vi "数据表比对.vi"(8 "error in (no error)":errorcluster, 9 "查询元素输入":string(combo), 10 "仪器日志参数":string, 11 "table输入":string(combo)) -> (0 "error out":errorcluster, 1 "columns输出":string[](array[string]), 2 "待发送第一条数据":string[](array[string]), 3 "待发送数据":string[][](table))   [LabVIEW 2016, in "数据传输系统.lvlib"]
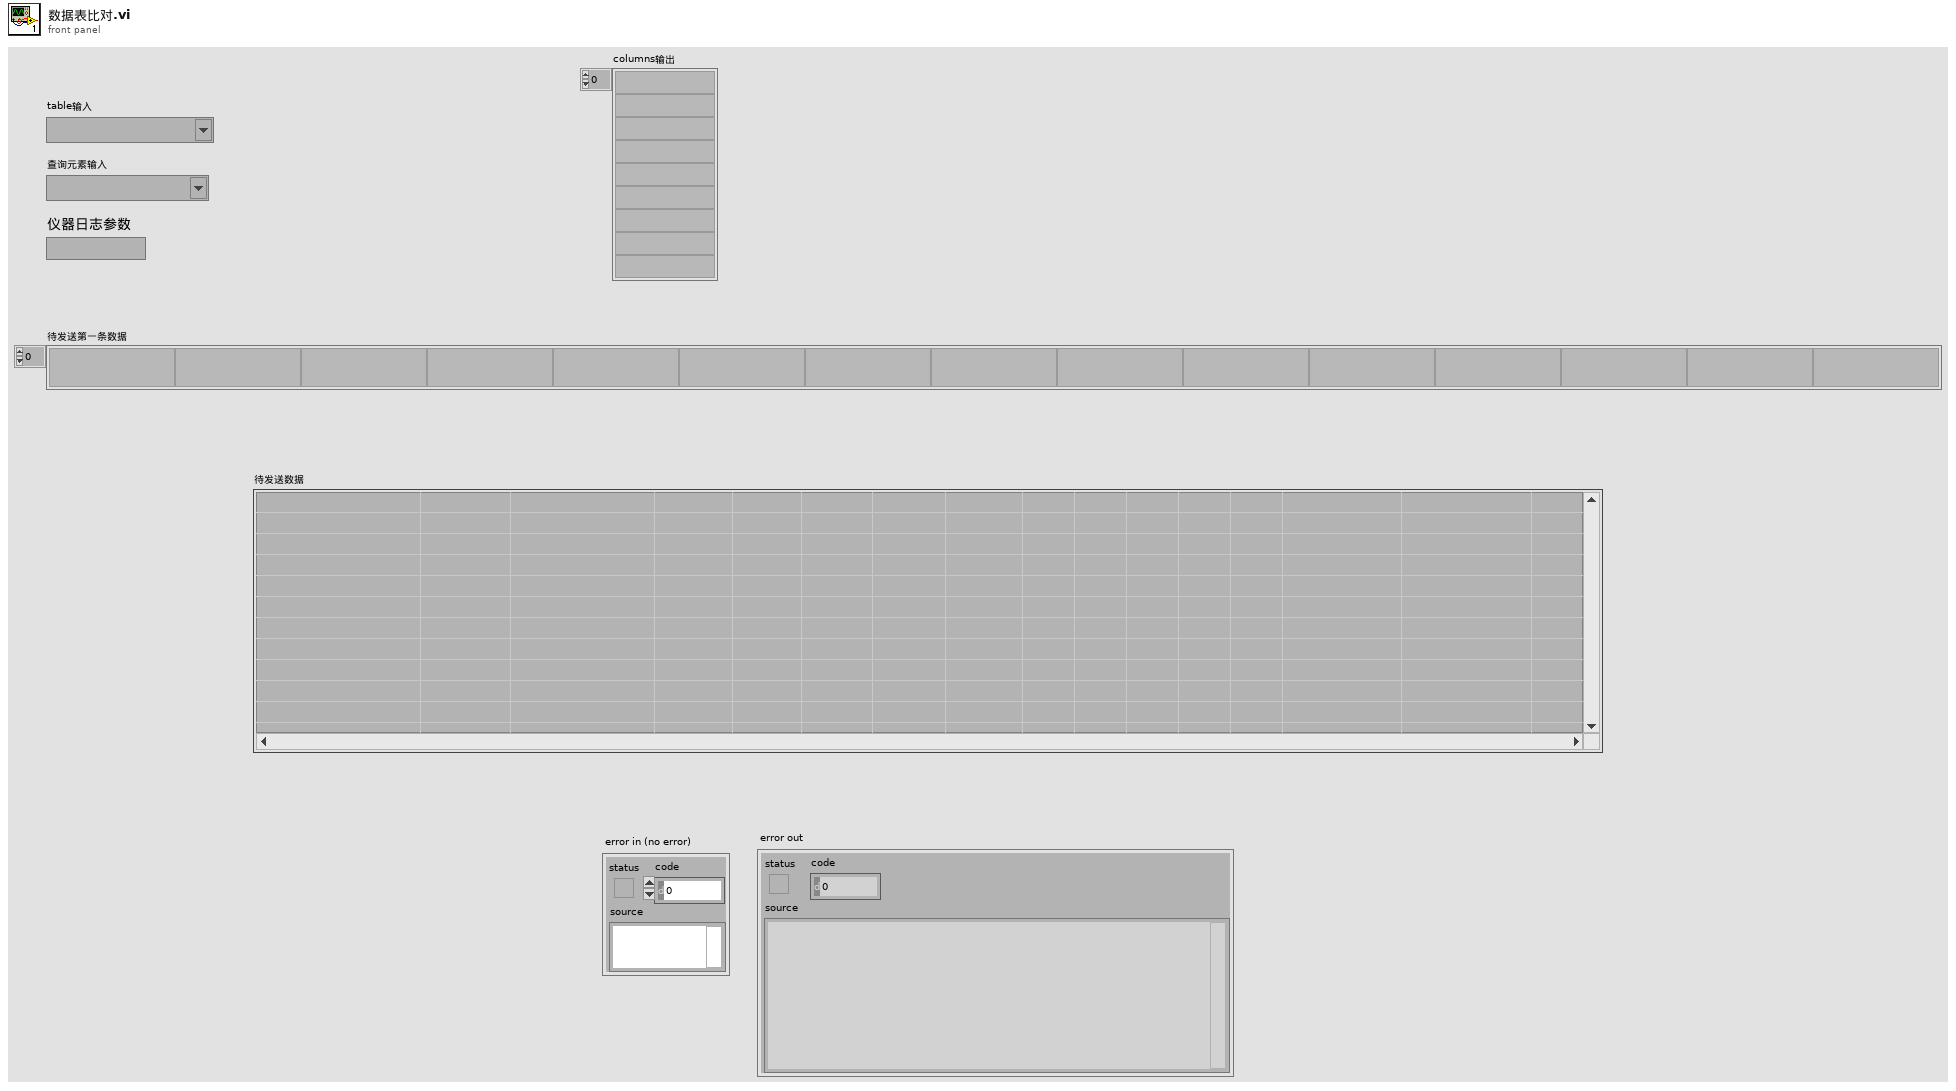
[diagram p1: front panel]
types:
  T1 = cluster{"氨氮仪器日志索引起始时间":string, "总磷仪器日志索引起始时间":string, "总氮仪器日志索引起始时间":string, "CODMn仪器日志索引起始时间":string, "CODCr仪器日志索引起始时间":string, "系统仪器日志索引起始时间":string}
  T2 = cluster{"氨氮仪器参数索引起始时间":string, "总磷仪器参数索引起始时间":string, "总氮仪器参数索引起始时间":string, "CODMn仪器参数索引起始时间":string, "CODCr仪器参数索引起始时间":string, "DO仪器参数索引起始时间":string, "PH仪器参数索引起始时间":string, "比电导率仪器参数索引起始时间":string, "水温仪器参数索引起始时间":string, "浊度仪器参数索引起始时间":string, "叶绿素a仪器参数索引起始时间":string, "藻密度仪器参数索引起始时间":string, "ORP仪器参数索引起始时间":string}
  T3 = cluster{"氨氮报警信息索引起始时间":string, "总磷报警信息索引起始时间":string, "总氮报警信息索引起始时间":string, "CODMn报警信息索引起始时间":string, "CODCr报警信息索引起始时间":string, "DO报警信息索引起始时间":string, "PH报警信息索引起始时间":string, "比电导率报警信息索引起始时间":string, "水温报警信息索引起始时间":string, "浊度报警信息索引起始时间":string, "叶绿素报警信息索引起始时间":string, "系统报警信息索引起始时间":string}
  T4 = cluster{"氨氮零点核查索引起始时间":string, "总磷零点核查索引起始时间":string, "总氮零点核查索引起始时间":string, "CODMn零点核查索引起始时间":string, "CODCr零点核查索引起始时间":string, "亚硝酸盐零点核查索引起始时间":string, "硫化物零点核查索引起始时间":string, "ORP零点核查索引起始时间":string}
  T5 = cluster{"氨氮标样核查索引起始时间":string, "总磷标样核查索引起始时间":string, "总氮标样核查索引起始时间":string, "CODMn标样核查索引起始时间":string, "CODCr标样核查索引起始时间":string, "DO标样核查索引起始时间":string, "PH标样核查索引起始时间":string, "比电导率标样核查索引起始时间":string, "水温标样核查索引起始时间":string, "浊度标样核查索引起始时间":string, "叶绿素a标样核查索引起始时间":string, "藻密度标样核查索引起始时间":string, "亚硝酸盐标样核查索引起始时间":string, "硫化物标样核查索引起始时间":string, "ORP标样核查索引起始时间":string}
  T6 = cluster{"氨氮跨度核查索引起始时间":string, "总磷跨度核查索引起始时间":string, "总氮跨度核查索引起始时间":string, "CODMn跨度核查索引起始时间":string, "CODCr跨度核查索引起始时间":string, "亚硝酸盐跨度核查索引起始时间":string, "硫化物跨度核查索引起始时间":string, "ORP跨度核查索引起始时间":string}
  T7 = typedef "LVDateTimeRec.ctl" = cluster{"秒数的小数部分":dbl, "秒":i32, "分":i32, "时":i32, "日":i32, "月":i32, "年":i32, "天数（周）":i32, "天数（年）":i32, "DST":i32}
  T8 = cluster{"氨氮加标回收索引起始时间":string, "总磷加标回收索引起始时间":string, "总氮加标回收索引起始时间":string, "CODMn加标回收索引起始时间":string, "CODCr加标回收索引起始时间":string}
  T9 = cluster{"氨氮平行样索引起始时间":string, "总磷平行样索引起始时间":string, "总氮平行样索引起始时间":string, "CODMn平行样索引起始时间":string, "CODCr平行样索引起始时间":string}
  T10 = cluster{"氨氮集成干预索引起始时间":string, "总磷集成干预索引起始时间":string, "总氮集成干预索引起始时间":string, "CODMn集成干预索引起始时间":string, "CODCr集成干预索引起始时间":string, "DO集成干预索引起始时间":string, "PH集成干预索引起始时间":string, "比电导率集成干预索引起始时间":string, "水温集成干预索引起始时间":string, "浊度集成干预索引起始时间":string, "叶绿素a集成干预索引起始时间":string, "藻密度集成干预索引起始时间":string, "亚硝酸盐集成干预索引起始时间":string, "硫化物集成干预索引起始时间":string, "ORP集成干预索引起始时间":string}
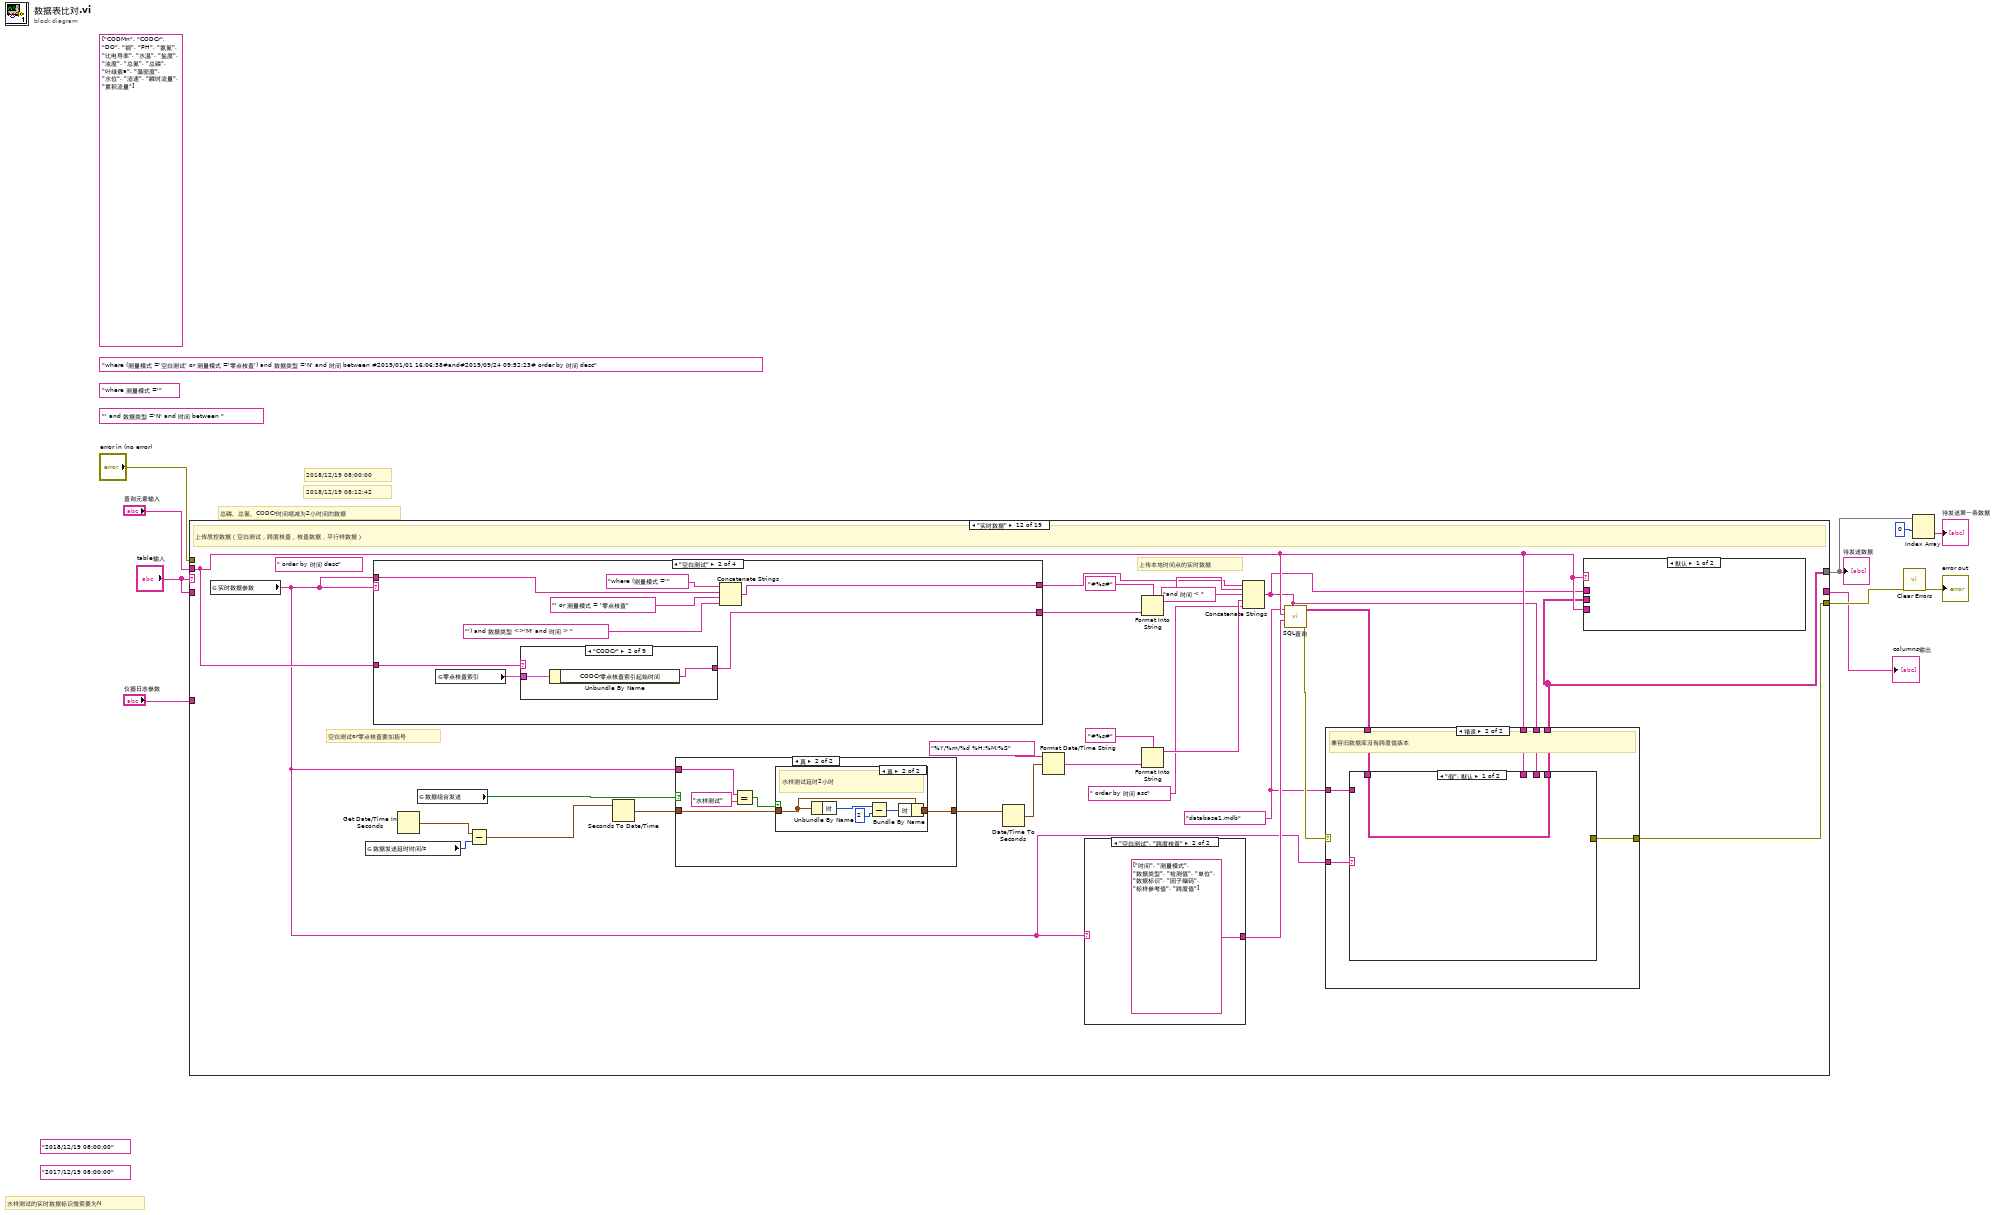
[diagram p0: block diagram]
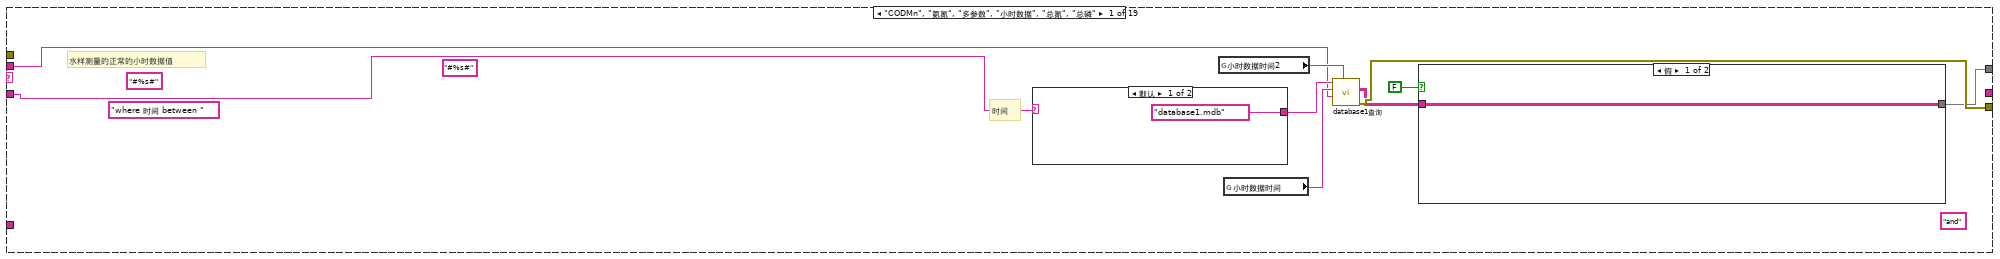
[diagram p2: hidden frame]
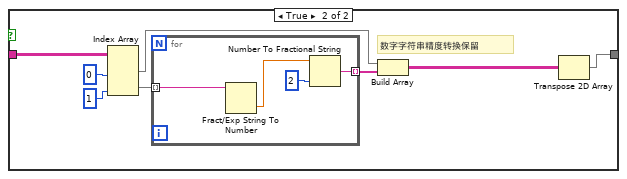
[diagram p3: hidden frame]
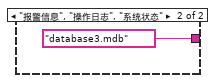
[diagram p4: hidden frame]
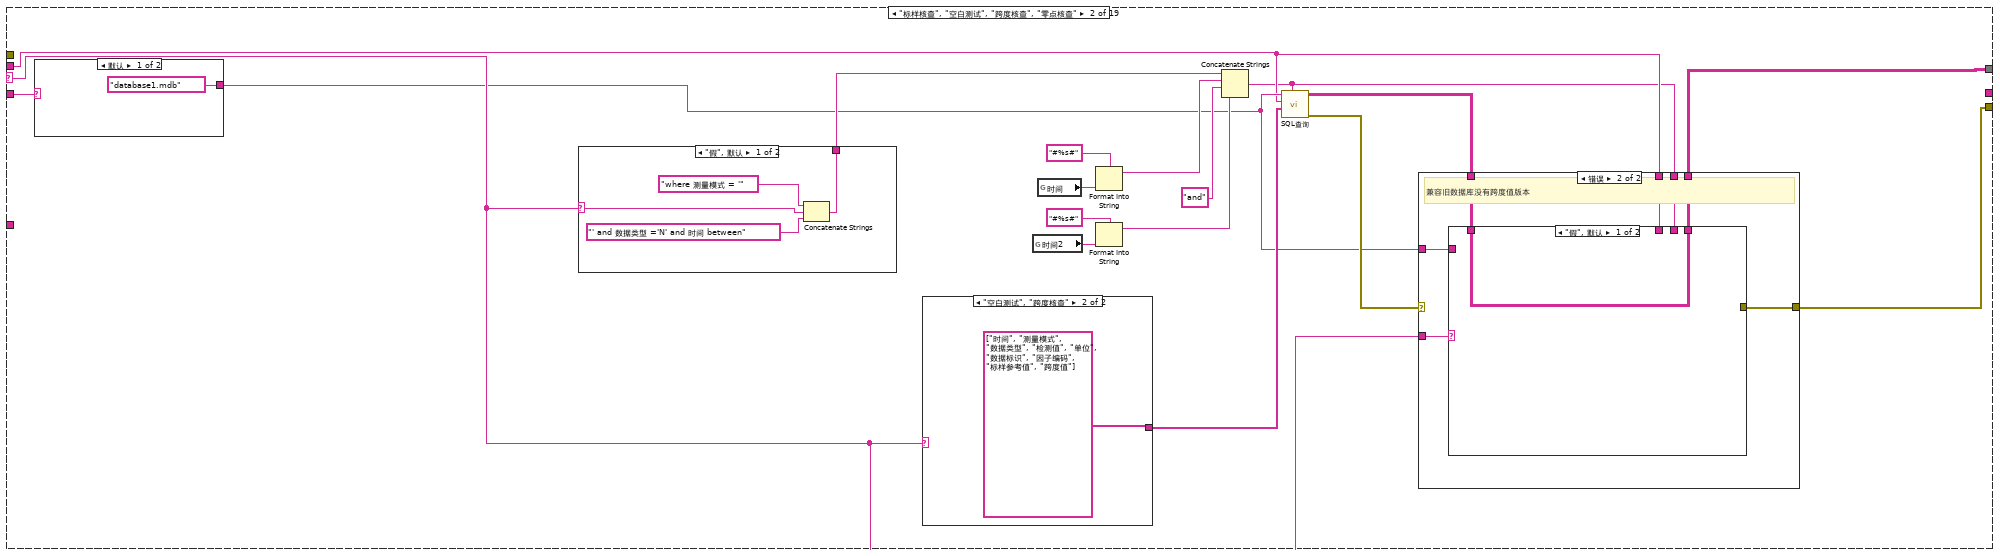
[diagram p5: hidden frame]
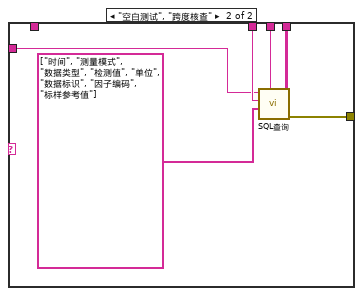
[diagram p7: hidden frame]
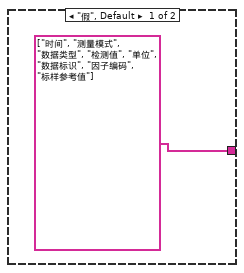
[diagram p8: hidden frame]
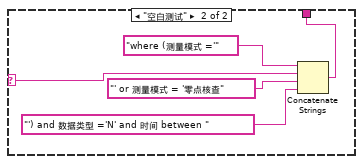
[diagram p9: hidden frame]
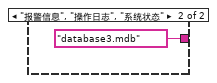
[diagram p10: hidden frame]
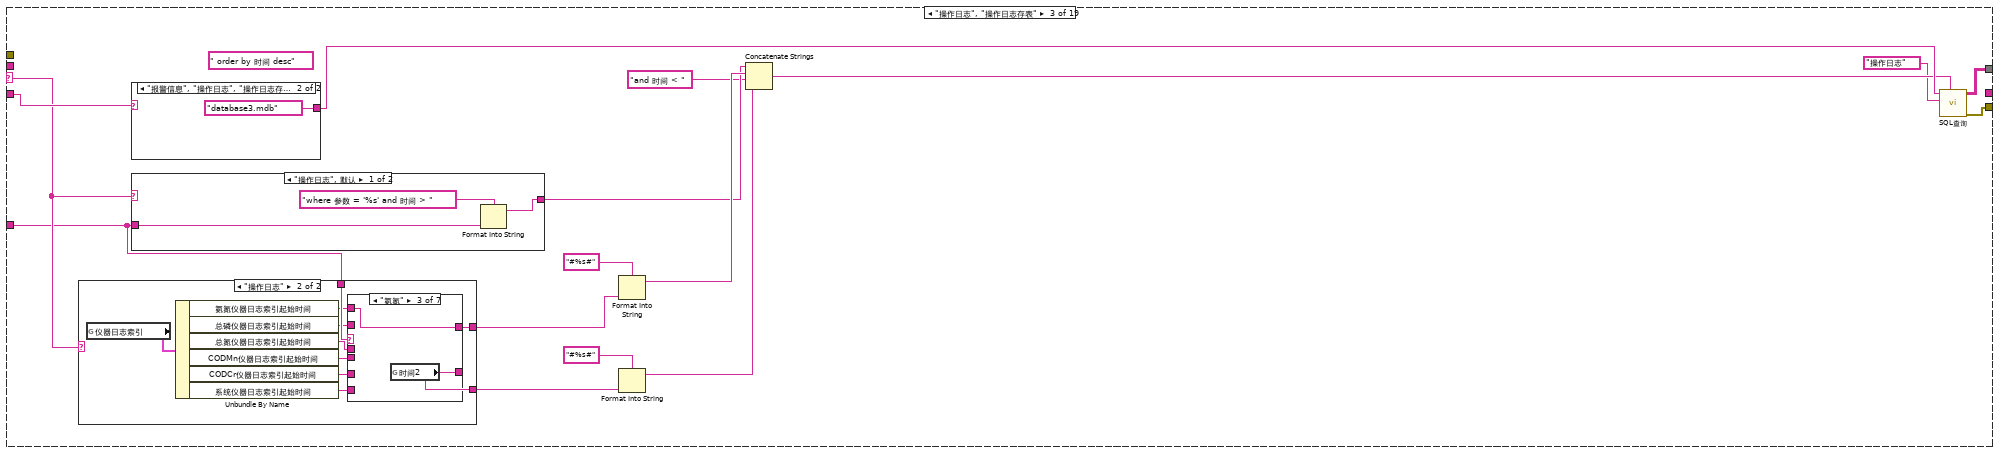
[diagram p11: hidden frame]
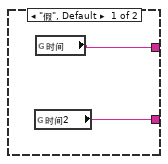
[diagram p12: hidden frame]
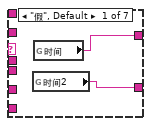
[diagram p13: hidden frame]
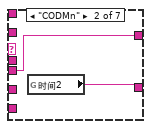
[diagram p14: hidden frame]
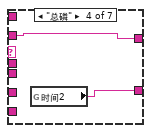
[diagram p15: hidden frame]
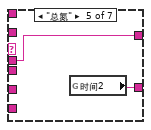
[diagram p16: hidden frame]
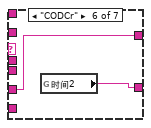
[diagram p17: hidden frame]
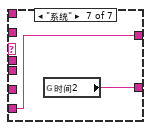
[diagram p18: hidden frame]
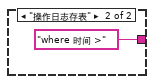
[diagram p19: hidden frame]
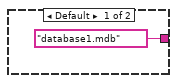
[diagram p20: hidden frame]
diagram:
  (unwired) "' and 数据类型 ='N' and 时间 between "
  (unwired) "where 测量模式 ='" ("condition")
  (unwired) "where (测量模式 ='空白测试' or 测量模式 ='零点核查') and 数据类型 ='N' and 时间 between #2019/01/01 16:06:38#and#2019/09/24 09:52:23# order by 时间 desc" ("condition")
  (unwired) string[] ["CODMn", "CODCr", "DO", "铜", "PH", "氨氮", "比电导率", "水温", "盐度", "浊度", "总氮", "总磷", "叶绿素a", "藻密度", "水位", "流速", "瞬时流量", "累积流量"] ("查询参数数组")
  (unwired) "2017/12/19 08:00:00"
  (unwired) "2018/12/19 08:00:00"
  # "水样测试的实时数据标识搜索要为N"
  # "2018/12/19 08:00:00"
  # "总磷、总氮、CODCr时间缩减为2小时间的数据"
  # "2018/12/19 08:12:42"
  n1 = case shown="\"实时数据\"" "table输入" {
    selector: "table输入" -> [_ w41 w86 _ _ _ _ w314 _ _ _ _ _ _ _ _ _ _ _]
    tunnel: "error in (no error)" -> [_ _ _ _ _ _ _ _ _ _ w418 _ _ _ _ _ _ _ _]
    tunnel: [w17 w35 w95 w144 w150 w202 w294 w328 w408 w415 w418 w419 w600 w661 w724 w788 w829 w872 w920] -> w8
    tunnel: [w13 w36 w93 w142 w178 w204 w286 w326 w387 w414 w416 w421 w603 w664 w722 w791 w832 w875 w922] -> w4
    tunnel: "table输入" -> [w19 w52 w97 _ w149 w205 _ w318 _ w411 _ _ _ _ _ _ _ _ _]
    tunnel: "查询元素输入" -> [w11 w39 _ _ _ _ _ _ _ _ _ w425 w590 w651 w710 w781 w822 w862 w916]
    tunnel: "仪器日志参数" -> [_ _ w83 w132 w170 w208 w275 w313 w396 _ _ _ _ _ _ _ _ _ _]
    tunnel: [_ _ _ _ _ _ _ _ _ w410 _ _ _ _ _ _ _ _ _] -> w1
    frame "CODMn", "氨氮", "多参数", "小时数据", "总氮", "总磷" {
      (unwired) "and" ("字符串")
      (unwired) "#%s#" ("初始字符串")
      (unwired) "#%s#" ("初始字符串")
      (unwired) "where 时间 between " ("condition")
      # "水样测量的正常的小时数据值"
      # "时间"
      n2 = case shown="默认" w19 {
        tunnel: ["database1.mdb" ("database") "database3.mdb" ("database")] -> w18
        frame Default {
        }
        frame "报警信息", "操作日志", "系统状态" {
        }
      }
      n3 = global read "全局 时间2.vi" "小时数据时间2"() -> (w15:string)
      n4 = global read "全局 水样时间.vi" "小时数据时间"() -> (w16:string)
      n5 = call "database1查询.vi"("时间2"=w15, "table"=w11, "时间1"=w16, "database"=w18) -> ("error out"=w17:errorcluster, "data"=w14:string[][])  [unwired: 4 in, 1 out]
      n6 = case shown="假" FALSE {
        tunnel: w14 -> [w20 w28]
        tunnel: [w20 w21] -> w13
        frame False {
        }
        frame True {
          # "数字字符串精度转换保留"
          n7 = Index Array(array=w28, index (col) #1=0 ("禁用的索引 (列)"), index (col) #2=1 ("索引 (列)")) -> (element #1=w24:string[], element #2=w25:string[])  [unwired: 2 in]
          n8 = for {
            tunnel: w25 -> [w30] mode=indexing
            tunnel: [w29] -> w23 mode=indexing
            n9 = Fract/Exp String To Number(string=w30) -> (number=w31:dbl)  [unwired: 3 in, 1 out]
            n10 = Number To Fractional String(number=w31, precision (6)=i16 2 ("精度(6)")) -> (F-format string=w29:string)  [unwired: 2 in]
          }
          n11 = Build Array(w24, w23) -> (w22:string[][])
          n12 = Transpose 2D Array(2D array=w22) -> (transposed array=w21:string[][])
        }
      }
    }
    frame "标样核查", "空白测试", "跨度核查", "零点核查" {
      n13 = case shown="默认" w52 {
        tunnel: ["database1.mdb" ("database") "database3.mdb" ("database")] -> w40
        frame Default {
        }
        frame "报警信息", "操作日志", "系统状态" {
        }
      }
      n14 = case shown="\"假\", 默认" w41 {
        selector: w41 -> [w73 w76]
        tunnel: [w71 w75] -> w44
        frame "假", Default {
          n15 = Concatenate Strings("where 测量模式 = '" ("condition"), w73, "' and 数据类型 ='N' and 时间 between" ("字符串")) -> (w71:string)
        }
        frame "空白测试" {
          n16 = Concatenate Strings("where (测量模式 ='" ("condition"), w76, "' or 测量模式 = '零点核查", "') and 数据类型 ='N' and 时间 between ") -> (w75:string)
        }
      }
      n17 = case shown="\"空白测试\", \"跨度核查\"" w41 {
        tunnel: [string[] ["时间", "测量模式", "数据类型", "检测值", "单位", "数据标识", "因子编码", "标样参考值"] ("columns") string[] ["时间", "测量模式", "数据类型", "检测值", "单位", "数据标识", "因子编码", "标样参考值", "跨度值"] ("columns")] -> w43
        frame "假", Default {
        }
        frame "空白测试", "跨度核查" {
        }
      }
      n18 = global read "全局 时间2.vi" "时间2"() -> (w45:string)
      n19 = global read "全局 水样时间.vi" "时间"() -> (w46:string)
      n20 = Format Into String(format string="#%s#" ("初始字符串"), w46) -> (resulting string=w51:string)  [unwired: 2 in, 1 out]
      n21 = Format Into String(format string="#%s#" ("初始字符串"), w45) -> (resulting string=w47:string)  [unwired: 2 in, 1 out]
      n22 = Concatenate Strings(w44, w51, "and" ("字符串"), w47) -> (w38:string)
      n23 = call "SQL查询.vi"("condition"=w38, "columns"=w43, "table输入"=w39, "database"=w40) -> ("error out"=w42:errorcluster, "data"=w37:string[][])  [unwired: 5 in, 1 out]
      n24 = case shown="错误" w42 {
        selector: w42 -> [w53 _]
        tunnel: w41 -> [_ w61]
        tunnel: w39 -> [_ w60]
        tunnel: w40 -> [_ w59]
        tunnel: w38 -> [_ w58]
        tunnel: w37 -> [w54 w56]
        tunnel: [w54 w57] -> w36
        tunnel: [w53 w55] -> w35
        frame No Error {
        }
        frame Error {
          # "兼容旧数据库没有跨度值版本"
          n25 = case shown="\"假\", 默认" w61 {
            tunnel: w60 -> [_ w67]
            tunnel: w59 -> [_ w66]
            tunnel: w58 -> [_ w65]
            tunnel: [w62 w64] -> w57
            tunnel: w56 -> [w62 _]
            tunnel: [_ w63] -> w55
            frame "假", Default {
            }
            frame "空白测试", "跨度核查" {
              n26 = call "SQL查询.vi"("condition"=w65, "columns"=string[] ["时间", "测量模式", "数据类型", "检测值", "单位", "数据标识", "因子编码", "标样参考值"], "table输入"=w67, "database"=w66) -> ("error out"=w63:errorcluster, "data"=w64:string[][])  [unwired: 5 in, 1 out]
            }
          }
        }
      }
    }
    frame "操作日志", "操作日志存表" {
      (unwired) " order by 时间 desc" ("字符串")
      n27 = case shown="\"操作日志\"" w86 {
        tunnel: [w99 w108] -> w85
        tunnel: [w98 w107] -> w84
        tunnel: w83 -> [_ w109]
        frame "假", Default {
          n28 = global read "全局 时间2.vi" "时间2"() -> (w98:string)
          n29 = global read "全局 水样时间.vi" "时间"() -> (w99:string)
        }
        frame "操作日志" {
          n30 = global read "全局 时间2.vi" "仪器日志索引"() -> (w106:T1)
          n31 = Unbundle By Name(w106) -> ("氨氮仪器日志索引起始时间"=w105:string, "总磷仪器日志索引起始时间"=w104:string, "总氮仪器日志索引起始时间"=w103:string, "CODMn仪器日志索引起始时间"=w102:string, "CODCr仪器日志索引起始时间"=w101:string, "系统仪器日志索引起始时间"=w100:string)
          n32 = case shown="\"氨氮\"" w109 {
            tunnel: [w110 w113 w115 w117 w119 w121 w123] -> w107
            tunnel: [w111 w112 w114 w116 w118 w120 w122] -> w108
            tunnel: w105 -> [_ _ w114 _ _ _ _]
            tunnel: w104 -> [_ _ _ w116 _ _ _]
            tunnel: w103 -> [_ _ _ _ w118 _ _]
            tunnel: w102 -> [_ w112 _ _ _ _ _]
            tunnel: w101 -> [_ _ _ _ _ w120 _]
            tunnel: w100 -> [_ _ _ _ _ _ w122]
            frame "假", Default {
              n33 = global read "全局 时间2.vi" "时间2"() -> (w110:string)
              n34 = global read "全局 水样时间.vi" "时间"() -> (w111:string)
            }
            frame "CODMn" {
              n35 = global read "全局 时间2.vi" "时间2"() -> (w113:string)
            }
            frame "氨氮" {
              n36 = global read "全局 时间2.vi" "时间2"() -> (w115:string)
            }
            frame "总磷" {
              n37 = global read "全局 时间2.vi" "时间2"() -> (w117:string)
            }
            frame "总氮" {
              n38 = global read "全局 时间2.vi" "时间2"() -> (w119:string)
            }
            frame "CODCr" {
              n39 = global read "全局 时间2.vi" "时间2"() -> (w121:string)
            }
            frame "系统" {
              n40 = global read "全局 时间2.vi" "时间2"() -> (w123:string)
            }
          }
        }
      }
      n41 = case shown="\"报警信息\", \"操作日志\", \"操作日志存表\", \"系统状态\"" w97 {
        tunnel: ["database1.mdb" ("database") "database3.mdb" ("database")] -> w96
        frame Default {
        }
        frame "报警信息", "操作日志", "操作日志存表", "系统状态" {
        }
      }
      n42 = case shown="\"操作日志\", 默认" w86 {
        tunnel: [w125 "where 时间 >" ("condition")] -> w88
        tunnel: w83 -> [w124 _]
        frame "操作日志", Default {
          n43 = Format Into String(format string="where 参数 = '%s' and 时间 > " ("condition"), w124) -> (resulting string=w125:string)  [unwired: 2 in, 1 out]
        }
        frame "操作日志存表" {
        }
      }
      n44 = Format Into String(format string="#%s#" ("初始字符串"), w85) -> (resulting string=w92:string)  [unwired: 2 in, 1 out]
      n45 = Format Into String(format string="#%s#" ("初始字符串"), w84) -> (resulting string=w89:string)  [unwired: 2 in, 1 out]
      n46 = Concatenate Strings(w88, w92, "and 时间 < " ("字符串"), w89) -> (w94:string)
      n47 = call "SQL查询.vi"("condition"=w94, "table输入"="操作日志", "database"=w96) -> ("error out"=w95:errorcluster, "data"=w93:string[][])  [unwired: 6 in, 1 out]
    }
    frame "提取操作日志" {
      (unwired) " order by 时间 desc" ("字符串")
      n48 = global read "全局 时间2.vi" "时间2"() -> (w133:string)
      n49 = global read "全局 水样时间.vi" "时间"() -> (w134:string)
      n50 = Format Into String(format string="where 参数 = '%s' and 时间 between" ("condition"), w132) -> (resulting string=w136:string)  [unwired: 2 in, 1 out]
      n51 = Format Into String(format string="#%s#" ("初始字符串"), w134) -> (resulting string=w141:string)  [unwired: 2 in, 1 out]
      n52 = Format Into String(format string="#%s#" ("初始字符串"), w133) -> (resulting string=w137:string)  [unwired: 2 in, 1 out]
      n53 = Concatenate Strings(w136, w141, "and" ("字符串"), w137) -> (w143:string)
      n54 = call "SQL查询.vi"("condition"=w143, "table输入"="操作日志", "database"="database3.mdb") -> ("error out"=w144:errorcluster, "data"=w142:string[][])  [unwired: 6 in, 1 out]
    }
    frame "3090仪器参数" {
      (unwired) string[] ["时间", "参数", "测量量程", "测量精度", "测量间隔", "消解温度", "消解时长", "空白校准时间", "曲线截距", "曲线斜率", "测量检出限", "测量信号值", "线性相关系数", "二次多项式系数", "标样校准时间", "稀释倍数", "三项式系数", "空白标定系数", "量程系数", "F0/ORPA", "F1/ORPB", "F2/ORPK", "F3", "F4", "F5", "F6", "F7", "X0/滴定数", "量程"] ("columns输出")
      n55 = case shown="\"仪器参数\", 默认" w149 {
        tunnel: [w181 w182] -> w165
        frame "3090仪器参数" {
          n56 = global read "全局 时间2.vi" "3090仪器参数索引"() -> (w181:T2)
        }
        frame "仪器参数", Default {
          n57 = global read "全局 时间2.vi" "仪器参数索引"() -> (w182:T2)
        }
      }
      n58 = Unbundle By Name(w165) -> ("氨氮仪器参数索引起始时间"=w164:string, "总磷仪器参数索引起始时间"=w163:string, "总氮仪器参数索引起始时间"=w162:string, "CODMn仪器参数索引起始时间"=w161:string, "CODCr仪器参数索引起始时间"=w160:string, "DO仪器参数索引起始时间"=w158:string, "PH仪器参数索引起始时间"=w157:string, "比电导率仪器参数索引起始时间"=w156:string, "水温仪器参数索引起始时间"=w155:string, "浊度仪器参数索引起始时间"=w154:string, "叶绿素a仪器参数索引起始时间"=w153:string, "藻密度仪器参数索引起始时间"=w152:string, "ORP仪器参数索引起始时间"=w151:string)
      n59 = global read "断电保存全局.vi" "数据发送延时时间/s"() -> (w146:i32)
      n60 = Get Date/Time In Seconds() -> (seconds since 1Jan1904=w147:timestamp)
      n61 = case shown="\"溶解氧\"" w170 {
        tunnel: w164 -> [_ _ w185 _ _ _ _ _ _ _ _ _ _ _]
        tunnel: w163 -> [_ _ _ w186 _ _ _ _ _ _ _ _ _ _]
        tunnel: w162 -> [_ _ _ _ w187 _ _ _ _ _ _ _ _ _]
        tunnel: w161 -> [w183 w184 _ _ _ _ _ _ _ _ _ _ _ _]
        tunnel: w160 -> [_ _ _ _ _ w188 _ _ _ _ _ _ _ _]
        tunnel: [w183 w184 w185 w186 w187 w188 w189 w190 w191 w192 w193 w194 w195 w196] -> w159
        tunnel: w158 -> [_ _ _ _ _ _ w189 _ _ _ _ _ _ _]
        tunnel: w157 -> [_ _ _ _ _ _ _ w190 _ _ _ _ _ _]
        tunnel: w156 -> [_ _ _ _ _ _ _ _ w191 _ _ _ _ _]
        tunnel: w155 -> [_ _ _ _ _ _ _ _ _ w192 _ _ _ _]
        tunnel: w154 -> [_ _ _ _ _ _ _ _ _ _ w193 _ _ _]
        tunnel: w153 -> [_ _ _ _ _ _ _ _ _ _ _ w194 _ _]
        tunnel: w152 -> [_ _ _ _ _ _ _ _ _ _ _ _ w195 _]
        tunnel: w151 -> [_ _ _ _ _ _ _ _ _ _ _ _ _ w196]
        frame "假", Default {
        }
        frame "CODMn" {
        }
        frame "氨氮" {
        }
        frame "总磷" {
        }
        frame "总氮" {
        }
        frame "CODCr" {
        }
        frame "溶解氧" {
        }
        frame "PH" {
        }
        frame "电导率" {
        }
        frame "水温" {
        }
        frame "浊度" {
        }
        frame "叶绿素" {
        }
        frame "藻密度" {
        }
        frame "ORP" {
        }
      }
      n62 = Subtract(x=w147, y=w146) -> (x-y=w145:timestamp)
      n63 = Format Date/Time String(time format string (%c)="%Y/%m/%d %H:%M:%S" ("时间格式字符串(%c)"), seconds (now)=w145) -> (date/time string=w168:string)  [unwired: 1 in]
      n64 = Search and Replace String(input string=w168, search string="." ("搜索字符串")) -> (result string=w166:string)  [unwired: 6 in, 3 out]
      n65 = Format Into String(format string="where 参数 = '%s' and 时间 > " ("condition"), w170) -> (resulting string=w173:string)  [unwired: 2 in, 1 out]
      n66 = Format Into String(format string="#%s#" ("初始字符串"), w159) -> (resulting string=w177:string)  [unwired: 2 in, 1 out]
      n67 = Format Into String(format string="#%s#" ("初始字符串"), w166) -> (resulting string=w174:string)  [unwired: 2 in, 1 out]
      n68 = Concatenate Strings(w173, w177, "and 时间 < " ("字符串"), w174, " order by 时间 asc" ("字符串")) -> (w179:string)
      n69 = call "SQL查询.vi"("condition"=w179, "table输入"=w149, "database"="database3.mdb") -> ("error out"=w150:errorcluster, "data"=w178:string[][])  [unwired: 6 in, 1 out]
    }
    frame "仪器参数" {
      n70 = case shown="\"仪器参数\", 默认" w205 {
        tunnel: [w254 w255] -> w225
        frame "3090仪器参数" {
          n71 = global read "全局 时间2.vi" "3090仪器参数索引"() -> (w254:T2)
        }
        frame "仪器参数", Default {
          n72 = global read "全局 时间2.vi" "仪器参数索引"() -> (w255:T2)
        }
      }
      n73 = Unbundle By Name(w225) -> ("氨氮仪器参数索引起始时间"=w224:string, "总磷仪器参数索引起始时间"=w223:string, "总氮仪器参数索引起始时间"=w222:string, "CODMn仪器参数索引起始时间"=w221:string, "CODCr仪器参数索引起始时间"=w220:string, "DO仪器参数索引起始时间"=w219:string, "PH仪器参数索引起始时间"=w218:string, "比电导率仪器参数索引起始时间"=w217:string, "水温仪器参数索引起始时间"=w216:string, "浊度仪器参数索引起始时间"=w215:string, "叶绿素a仪器参数索引起始时间"=w214:string, "藻密度仪器参数索引起始时间"=w213:string, "ORP仪器参数索引起始时间"=w212:string)
      n74 = Get Date/Time In Seconds() -> (seconds since 1Jan1904=w198:timestamp)
      n75 = global read "断电保存全局.vi" "数据发送延时时间/s"() -> (w199:i32)
      n76 = case shown="\"溶解氧\"" w208 {
        tunnel: w224 -> [_ _ w258 _ _ _ _ _ _ _ _ _ _ _]
        tunnel: w223 -> [_ _ _ w259 _ _ _ _ _ _ _ _ _ _]
        tunnel: w222 -> [_ _ _ _ w260 _ _ _ _ _ _ _ _ _]
        tunnel: w221 -> [w256 w257 _ _ _ _ _ _ _ _ _ _ _ _]
        tunnel: w220 -> [_ _ _ _ _ w261 _ _ _ _ _ _ _ _]
        tunnel: [w256 w257 w258 w259 w260 w261 w262 w263 w264 w265 w266 w267 w268 w269] -> w207
        tunnel: w219 -> [_ _ _ _ _ _ w262 _ _ _ _ _ _ _]
        tunnel: w218 -> [_ _ _ _ _ _ _ w263 _ _ _ _ _ _]
        tunnel: w217 -> [_ _ _ _ _ _ _ _ w264 _ _ _ _ _]
        tunnel: w216 -> [_ _ _ _ _ _ _ _ _ w265 _ _ _ _]
        tunnel: w215 -> [_ _ _ _ _ _ _ _ _ _ w266 _ _ _]
        tunnel: w214 -> [_ _ _ _ _ _ _ _ _ _ _ w267 _ _]
        tunnel: w213 -> [_ _ _ _ _ _ _ _ _ _ _ _ w268 _]
        tunnel: w212 -> [_ _ _ _ _ _ _ _ _ _ _ _ _ w269]
        frame "假", Default {
        }
        frame "CODMn" {
        }
        frame "氨氮" {
        }
        frame "总磷" {
        }
        frame "总氮" {
        }
        frame "CODCr" {
        }
        frame "溶解氧" {
        }
        frame "PH" {
        }
        frame "电导率" {
        }
        frame "水温" {
        }
        frame "浊度" {
        }
        frame "叶绿素" {
        }
        frame "藻密度" {
        }
        frame "ORP" {
        }
      }
      n77 = Subtract(x=w198, y=w199) -> (x-y=w197:timestamp)
      n78 = Format Date/Time String(time format string (%c)="%Y/%m/%d %H:%M:%S" ("时间格式字符串(%c)"), seconds (now)=w197) -> (date/time string=w227:string)  [unwired: 1 in]
      n79 = Search and Replace String(input string=w227, search string="." ("搜索字符串")) -> (result string=w206:string)  [unwired: 6 in, 3 out]
      n80 = Format Into String(format string="#%s#" ("初始字符串"), w206) -> (resulting string=w230:string)  [unwired: 2 in, 1 out]
      n81 = Format Into String(format string="#%s#" ("初始字符串"), w207) -> (resulting string=w233:string)  [unwired: 2 in, 1 out]
      n82 = Concatenate Strings("where 数据类型 ='N' and 时间 > " ("condition"), w233, "and 时间 < " ("字符串"), w230, " order by 时间 asc" ("字符串")) -> (w234:string)
      n83 = call "SQL查询.vi"("condition"=w234, "columns"=string[] ["时间", "数据类型", "测量量程", "测量精度", "测量间隔", "消解温度", "消解时长", "空白校准时间", "曲线截距", "曲线斜率", "测量检出限", "测量信号值", "线性相关系数", "二次多项式系数", "标样校准时间"] ("columns输出"), "table输入"=w208, "database"="database1.mdb") -> ("error out"=w201:errorcluster, "data"=w203:string[][])  [unwired: 5 in, 1 out]
      n84 = Empty Array?(array=w203) -> (empty?=w209:bool)
      n85 = case shown="假" w209 {
        tunnel: w208 -> [_ w251]
        tunnel: w207 -> [_ w247]
        tunnel: w206 -> [_ w243]
        tunnel: w205 -> [_ w240]
        tunnel: [w237 w239] -> w204
        tunnel: w203 -> [w237 _]
        tunnel: [w236 w238] -> w202
        tunnel: w201 -> [w236 _]
        frame False {
        }
        frame True {
          n86 = Format Into String(format string="#%s#" ("初始字符串"), w247) -> (resulting string=w246:string)  [unwired: 2 in, 1 out]
          n87 = Format Into String(format string="#%s#" ("初始字符串"), w243) -> (resulting string=w242:string)  [unwired: 2 in, 1 out]
          n88 = Format Into String(format string="where 参数 = '%s' and 时间 between" ("condition"), w251) -> (resulting string=w249:string)  [unwired: 2 in, 1 out]
          n89 = Concatenate Strings(w249, w246, "and" ("字符串"), w242, " order by 时间 asc" ("字符串")) -> (w250:string)
          n90 = call "SQL查询.vi"("condition"=w250, "table输入"=w240, "database"="database3.mdb") -> ("error out"=w238:errorcluster, "data"=w239:string[][])  [unwired: 6 in, 1 out]
        }
      }
    }
    frame "提取仪器参数" {
      w288 = 0 ("索引 (行)")
      n91 = global read "全局 水样时间.vi" "时间"() -> (w277:string)
      n92 = global read "全局 时间2.vi" "时间2"() -> (w279:string)
      n93 = Format Into String(format string="#%s#" ("初始字符串"), w277) -> (resulting string=w284:string)  [unwired: 2 in, 1 out]
      n94 = Format Into String(format string="#%s#" ("初始字符串"), w279) -> (resulting string=w280:string)  [unwired: 2 in, 1 out]
      n95 = Concatenate Strings("where 数据类型 ='N' and 时间 between" ("condition"), w284, "and" ("字符串"), w280, " order by 时间 desc" ("字符串")) -> (w276:string)
      n96 = call "SQL查询.vi"("condition"=w276, "columns"=string[] ["时间", "数据类型", "测量量程", "测量精度", "测量间隔", "消解温度", "消解时长", "空白校准时间", "曲线截距", "曲线斜率", "测量检出限", "测量信号值", "线性相关系数", "二次多项式系数", "标样校准时间"] ("columns输出"), "table输入"=w275, "database"="database1.mdb") -> ("error out"=w272:errorcluster, "data"=w273:string[][])  [unwired: 5 in, 1 out]
      n97 = Empty Array?(array=w273) -> (empty?=w274:bool)
      n98 = case shown="真" w274 {
        tunnel: [w295 w311] -> w294
        tunnel: w275 -> [_ w299]
        tunnel: [w296 w297] -> w293
        tunnel: w273 -> [w296 _]
        tunnel: w272 -> [w295 _]
        frame False {
        }
        frame True {
          n99 = global read "全局 水样时间.vi" "时间"() -> (w298:string)
          n100 = global read "全局 时间2.vi" "时间2"() -> (w304:string)
          n101 = Format Into String(format string="where 参数 = '%s' and 时间 between" ("condition"), w299) -> (resulting string=w303:string)  [unwired: 2 in, 1 out]
          n102 = Format Into String(format string="#%s#" ("初始字符串"), w298) -> (resulting string=w309:string)  [unwired: 2 in, 1 out]
          n103 = Format Into String(format string="#%s#" ("初始字符串"), w304) -> (resulting string=w305:string)  [unwired: 2 in, 1 out]
          n104 = Concatenate Strings(w303, w309, "and" ("字符串"), w305, " order by 时间 desc" ("字符串")) -> (w310:string)
          n105 = call "SQL查询.vi"("condition"=w310, "table输入"="仪器参数", "database"="database3.mdb") -> ("error out"=w311:errorcluster, "data"=w297:string[][])  [unwired: 6 in, 1 out]
        }
      }
      n106 = Get Date/Time In Seconds() -> (seconds since 1Jan1904=w290:timestamp)
      n107 = Format Date/Time String(time format string (%c)="%Y/%m/%d %H:%M:%S" ("时间格式字符串(%c)"), seconds (now)=w290) -> (date/time string=w291:string)  [unwired: 1 in]
      n108 = Search and Replace String(input string=w291, search string="." ("搜索字符串")) -> (result string=w287:string)  [unwired: 6 in, 3 out]
      n109 = Replace Array Subset(array=w293, new element=w287, index (row)=w288, index (col)=w288) -> (w286:string[][])
    }
    frame "报警信息", "报警信息存表" {
      # "时间"
      n110 = case shown="\"\", 默认" w314 {
        tunnel: [w331 w334] -> w315
        tunnel: [w330 w333] -> w316
        tunnel: w313 -> [_ w335]
        frame "", Default {
          n111 = global read "全局 时间2.vi" "时间2"() -> (w330:string)
          n112 = global read "全局 水样时间.vi" "时间"() -> (w331:string)
        }
        frame "报警信息" {
          n113 = global read "全局 时间2.vi" "报警信息索引"() -> (w332:T3)
          n114 = case shown="\"系统\"" w335 {
            tunnel: [w336 w340 w343 w346 w349 w352 w355 w358 w361 w364 w367 w370 w373] -> w333
            tunnel: [w337 w339 w341 w344 w347 w350 w353 w356 w359 w362 w365 w368 w371] -> w334
            tunnel: w332 -> [_ w338 w342 w345 w348 w351 w354 w357 w360 w363 w366 w369 w372]
            frame "假", Default {
              n115 = global read "全局 时间2.vi" "时间2"() -> (w336:string)
              n116 = global read "全局 水样时间.vi" "时间"() -> (w337:string)
            }
            frame "CODMn" {
              n117 = Unbundle By Name(w338) -> ("CODMn报警信息索引起始时间"=w339:string)
              n118 = global read "全局 时间2.vi" "时间2"() -> (w340:string)
            }
            frame "氨氮" {
              n119 = Unbundle By Name(w342) -> ("氨氮报警信息索引起始时间"=w341:string)
              n120 = global read "全局 时间2.vi" "时间2"() -> (w343:string)
            }
            frame "总磷" {
              n121 = Unbundle By Name(w345) -> ("总磷报警信息索引起始时间"=w344:string)
              n122 = global read "全局 时间2.vi" "时间2"() -> (w346:string)
            }
            frame "总氮" {
              n123 = Unbundle By Name(w348) -> ("总氮报警信息索引起始时间"=w347:string)
              n124 = global read "全局 时间2.vi" "时间2"() -> (w349:string)
            }
            frame "CODCr" {
              n125 = Unbundle By Name(w351) -> ("CODCr报警信息索引起始时间"=w350:string)
              n126 = global read "全局 时间2.vi" "时间2"() -> (w352:string)
            }
            frame "DO" {
              n127 = Unbundle By Name(w354) -> ("DO报警信息索引起始时间"=w353:string)
              n128 = global read "全局 时间2.vi" "时间2"() -> (w355:string)
            }
            frame "PH" {
              n129 = Unbundle By Name(w357) -> ("PH报警信息索引起始时间"=w356:string)
              n130 = global read "全局 时间2.vi" "时间2"() -> (w358:string)
            }
            frame "电导率" {
              n131 = Unbundle By Name(w360) -> ("比电导率报警信息索引起始时间"=w359:string)
              n132 = global read "全局 时间2.vi" "时间2"() -> (w361:string)
            }
            frame "水温" {
              n133 = Unbundle By Name(w363) -> ("水温报警信息索引起始时间"=w362:string)
              n134 = global read "全局 时间2.vi" "时间2"() -> (w364:string)
            }
            frame "浊度" {
              n135 = Unbundle By Name(w366) -> ("浊度报警信息索引起始时间"=w365:string)
              n136 = global read "全局 时间2.vi" "时间2"() -> (w367:string)
            }
            frame "叶绿素" {
              n137 = Unbundle By Name(w369) -> ("叶绿素报警信息索引起始时间"=w368:string)
              n138 = global read "全局 时间2.vi" "时间2"() -> (w370:string)
            }
            frame "系统" {
              n139 = Unbundle By Name(w372) -> ("系统报警信息索引起始时间"=w371:string)
              n140 = global read "全局 时间2.vi" "时间2"() -> (w373:string)
            }
          }
        }
      }
      n141 = case shown="\"环境参数\"" w314 {
        tunnel: [" order by 时间 desc" ("字符串") "" ("仪器日志参数")] -> w317
        frame "环境参数" {
        }
        frame "报警信息", Default {
        }
      }
      n142 = case shown="\"报警信息\", \"报警信息存表\", \"操作日志\", \"系统状态\"" w318 {
        tunnel: ["database1.mdb" ("database") "database3.mdb" ("database")] -> w329
        frame Default {
        }
        frame "报警信息", "报警信息存表", "操作日志", "系统状态" {
        }
      }
      n143 = case shown="\"报警信息\", 默认" w318 {
        tunnel: [w376 "报警信息" ("table输入")] -> w319
        frame "环境参数" {
          n144 = local read "仪器日志参数"() -> (w376:string)
        }
        frame "报警信息", Default {
        }
      }
      n145 = case shown="\"报警信息\", 默认" w314 {
        tunnel: [w379 w382 "where 时间 between" ("condition")] -> w320
        tunnel: w313 -> [w378 w381 _]
        frame "报警信息", Default {
          n146 = Format Into String(format string="where 参数 = '%s' and 时间 between" ("condition"), w378) -> (resulting string=w379:string)  [unwired: 2 in, 1 out]
        }
        frame "环境参数" {
          n147 = Format Into String(format string="where 参数 = '%s' and 时间 between" ("condition"), w381) -> (resulting string=w382:string)  [unwired: 2 in, 1 out]
        }
        frame "报警信息存表" {
        }
      }
      n148 = Format Into String(format string="#%s#" ("初始字符串"), w315) -> (resulting string=w325:string)  [unwired: 2 in, 1 out]
      n149 = Format Into String(format string="#%s#" ("初始字符串"), w316) -> (resulting string=w321:string)  [unwired: 2 in, 1 out]
      n150 = Concatenate Strings(w320, w325, "and" ("字符串"), w321, w317) -> (w327:string)
      n151 = call "SQL查询.vi"("condition"=w327, "table输入"=w319, "database"=w329) -> ("error out"=w328:errorcluster, "data"=w326:string[][])  [unwired: 6 in, 1 out]
    }
    frame "提取报警信息" {
      w390 = 0 ("索引 (行)")
      # "时间"
      # "提取仪器状态"
      n152 = global read "全局 水样时间.vi" "时间"() -> (w397:string)
      n153 = global read "全局 时间2.vi" "时间2"() -> (w398:string)
      n154 = Format Into String(format string="where 参数 = '%s' and 时间 between" ("condition"), w396) -> (resulting string=w401:string)  [unwired: 2 in, 1 out]
      n155 = Format Into String(format string="#%s#" ("初始字符串"), w397) -> (resulting string=w406:string)  [unwired: 2 in, 1 out]
      n156 = Format Into String(format string="#%s#" ("初始字符串"), w398) -> (resulting string=w402:string)  [unwired: 2 in, 1 out]
      n157 = Concatenate Strings(w401, w406, "and" ("字符串"), w402, " order by 时间 desc" ("仪器日志参数")) -> (w407:string)
      n158 = Get Date/Time In Seconds() -> (seconds since 1Jan1904=w392:timestamp)
      n159 = Format Date/Time String(time format string (%c)="%Y/%m/%d %H:%M:%S" ("时间格式字符串(%c)"), seconds (now)=w392) -> (date/time string=w393:string)  [unwired: 1 in]
      n160 = call "SQL查询.vi"("condition"=w407, "table输入"="报警信息", "database"="database3.mdb") -> ("error out"=w408:errorcluster, "data"=w388:string[][])  [unwired: 6 in, 1 out]
      n161 = Search and Replace String(input string=w393, search string="." ("搜索字符串")) -> (result string=w389:string)  [unwired: 6 in, 3 out]
      n162 = Replace Array Subset(array=w388, new element=w389, index (row)=w390, index (col)=w390) -> (w387:string[][])
    }
    frame "环境参数" {
      n163 = call "SQL查询.vi"("condition"=" order by 时间 desc" ("字符串"), "table输入"=w411, "database"="database1.mdb") -> ("error out"=w415:errorcluster, "columns输出"=w410:string[], "data"=w414:string[][])  [unwired: 6 in]
    }
    frame Default {
      # "时间格式转换"
      n164 = local read "待发送数据"() -> (w417:string[][])
      n165 = call "数组时间戳格式化(子VI).vi"("待发送数据输入"=w417) -> ("待发送数据输出"=w416:string[][])  [unwired: 10 in]
    }
    frame "实时数据" {
      (unwired) " order by 时间 desc" ("字符串")
      w424 = "database1.mdb" ("database")
      # "空白测试or零点核查要加括号"
      # "上传本地时间点的实时数据"
      # "上传质控数据（空白测试，跨度核查，核查数据，平行样数据）"
      n166 = global read "全局 实时数据参数.vi" "实时数据参数"() -> (w420:string)
      n167 = global read "断电保存全局.vi" "数据发送延时时间/s"() -> (w429:i32)
      n168 = case shown="\"空白测试\"" w420 {
        tunnel: [w479 w502 w521 w558] -> w439
        tunnel: w420 -> [w475 w501 _ w562]
        tunnel: [w478 w497 w523 w561] -> w435
        tunnel: w425 -> [_ w496 _ _]
        frame "水样测试" {
          n169 = Get Date/Time In Seconds() -> (seconds since 1Jan1904=w487:timestamp)
          n170 = Format Date/Time String(time format string (%c)="%Y%m%d%H%M%S%3u" ("时间格式字符串(%c)"), seconds (now)=w487) -> (date/time string=w485:string)  [unwired: 1 in]
          n171 = local read "查询元素输入"() -> (w480:string)
          n172 = Concatenate Strings("where 测量模式 ='" ("condition"), w475, "' and 数据类型 ='N' and 时间 > ") -> (w478:string)
          n173 = Replace Substring(2:8 ("长度（子字符串长度）"), 3:10 ("偏移量(0)"), 4:"0000" ("子字符串(\"\")"), 5:w485) -> (1:w481:string)  [unwired: 1 out]
          n174 = case shown="\"CODCr加标回收率\", \"CODMn加标回收率\", \"氨氮加标回收率\", \"总氮加标回收率\", \"总磷加标回收率\"" w480 {
            tunnel: w481 -> [w489 w492 _]
            tunnel: [w488 w493 w494] -> w479
            frame Default {
              n175 = Search and Replace String(input string=w489, search string="." ("搜索字符串")) -> (result string=w490:string)  [unwired: 6 in, 3 out]
              n176 = call "格式时间字符串.vi"("字符串"=w490) -> ("连接的字符串"=w488:string)  [unwired: 10 in]
            }
            frame "CODCr", "CODMn", "累积流量", "总氮", "总磷" {
              n177 = call "实时数据查询用2小时间的数据.vi"("字符串"=w492) -> ("连接的字符串"=w493:string)  [unwired: 10 in]
            }
            frame "CODCr加标回收率", "CODMn加标回收率", "氨氮加标回收率", "总氮加标回收率", "总磷加标回收率" {
              n178 = global read "全局 时间2.vi" "加标回收索引起始时间"() -> (w494:string)
            }
          }
        }
        frame "空白测试" {
          n179 = global read "全局 时间2.vi" "零点核查索引"() -> (w495:T4)
          n180 = case shown="\"CODCr\"" w496 {
            tunnel: [w503 w505 w507 w509 w511 w514 w515 w517 w519] -> w502
            tunnel: w495 -> [w504 w506 w508 w510 w512 w513 w516 w518 _]
            frame "CODMn" {
              n181 = Unbundle By Name(w504) -> ("CODMn零点核查索引起始时间"=w503:string)
            }
            frame "CODCr" {
              n182 = Unbundle By Name(w506) -> ("CODCr零点核查索引起始时间"=w505:string)
            }
            frame "氨氮" {
              n183 = Unbundle By Name(w508) -> ("氨氮零点核查索引起始时间"=w507:string)
            }
            frame "总磷" {
              n184 = Unbundle By Name(w510) -> ("总磷零点核查索引起始时间"=w509:string)
            }
            frame "总氮" {
              n185 = Unbundle By Name(w512) -> ("总氮零点核查索引起始时间"=w511:string)
            }
            frame "亚硝酸盐" {
              n186 = Unbundle By Name(w513) -> ("亚硝酸盐零点核查索引起始时间"=w514:string)
            }
            frame "硫化物" {
              n187 = Unbundle By Name(w516) -> ("硫化物零点核查索引起始时间"=w515:string)
            }
            frame "ORP" {
              n188 = Unbundle By Name(w518) -> ("ORP零点核查索引起始时间"=w517:string)
            }
            frame "", Default {
              n189 = global read "全局 时间2.vi" "零点核查索引起始时间"() -> (w519:string)
            }
          }
          n190 = Concatenate Strings("where (测量模式 ='" ("condition"), w501, "' or 测量模式 = '零点核查", "') and 数据类型 <>'M' and 时间 > ") -> (w497:string)
        }
        frame "核查数据" {
          n191 = local read "查询元素输入"() -> (w522:string)
          n192 = global read "全局 时间2.vi" "标样核查索引"() -> (w520:T5)
          n193 = case shown="\"ORP\"" w522 {
            tunnel: [w527 w529 w531 w533 w535 w537 w539 w541 w543 w545 w547 w549 w551 w553 w555 w557] -> w521
            tunnel: w520 -> [w528 w530 w532 w534 w536 w538 w540 w542 w544 w546 w548 w550 w552 w554 w556 _]
            frame "CODMn" {
              n194 = Unbundle By Name(w528) -> ("CODMn标样核查索引起始时间"=w527:string)
            }
            frame "CODCr" {
              n195 = Unbundle By Name(w530) -> ("CODCr标样核查索引起始时间"=w529:string)
            }
            frame "氨氮" {
              n196 = Unbundle By Name(w532) -> ("氨氮标样核查索引起始时间"=w531:string)
            }
            frame "总磷" {
              n197 = Unbundle By Name(w534) -> ("总磷标样核查索引起始时间"=w533:string)
            }
            frame "总氮" {
              n198 = Unbundle By Name(w536) -> ("总氮标样核查索引起始时间"=w535:string)
            }
            frame "DO" {
              n199 = Unbundle By Name(w538) -> ("DO标样核查索引起始时间"=w537:string)
            }
            frame "PH" {
              n200 = Unbundle By Name(w540) -> ("PH标样核查索引起始时间"=w539:string)
            }
            frame "比电导率" {
              n201 = Unbundle By Name(w542) -> ("比电导率标样核查索引起始时间"=w541:string)
            }
            frame "水温" {
              n202 = Unbundle By Name(w544) -> ("水温标样核查索引起始时间"=w543:string)
            }
            frame "浊度" {
              n203 = Unbundle By Name(w546) -> ("浊度标样核查索引起始时间"=w545:string)
            }
            frame "叶绿素a" {
              n204 = Unbundle By Name(w548) -> ("叶绿素a标样核查索引起始时间"=w547:string)
            }
            frame "藻密度" {
              n205 = Unbundle By Name(w550) -> ("藻密度标样核查索引起始时间"=w549:string)
            }
            frame "亚硝酸盐" {
              n206 = Unbundle By Name(w552) -> ("亚硝酸盐标样核查索引起始时间"=w551:string)
            }
            frame "硫化物" {
              n207 = Unbundle By Name(w554) -> ("硫化物标样核查索引起始时间"=w553:string)
            }
            frame "ORP" {
              n208 = Unbundle By Name(w556) -> ("ORP标样核查索引起始时间"=w555:string)
            }
            frame "", Default {
              n209 = global read "全局 时间2.vi" "标样核查索引起始时间"() -> (w557:string)
            }
          }
          n210 = Concatenate Strings("where 测量模式 ='" ("condition"), "标样核查" ("实时数据参数"), "' and 数据类型 <>'M' and 时间 > ") -> (w523:string)
        }
        frame "跨度核查", Default {
          n211 = local read "查询元素输入"() -> (w559:string)
          n212 = global read "全局 时间2.vi" "跨度核查索引"() -> (w560:T6)
          n213 = Concatenate Strings("where 测量模式 ='" ("condition"), w562, "' and 数据类型 <>'M' and 时间 > ") -> (w561:string)
          n214 = case shown="\"氨氮\"" w559 {
            tunnel: [w565 w567 w569 w571 w573 w576 w577 w579 w581] -> w558
            tunnel: w560 -> [w566 w568 w570 w572 w574 w575 w578 w580 _]
            frame "CODMn" {
              n215 = Unbundle By Name(w566) -> ("CODMn跨度核查索引起始时间"=w565:string)
            }
            frame "CODCr" {
              n216 = Unbundle By Name(w568) -> ("CODCr跨度核查索引起始时间"=w567:string)
            }
            frame "氨氮" {
              n217 = Unbundle By Name(w570) -> ("氨氮跨度核查索引起始时间"=w569:string)
            }
            frame "总磷" {
              n218 = Unbundle By Name(w572) -> ("总磷跨度核查索引起始时间"=w571:string)
            }
            frame "总氮" {
              n219 = Unbundle By Name(w574) -> ("总氮跨度核查索引起始时间"=w573:string)
            }
            frame "亚硝酸盐" {
              n220 = Unbundle By Name(w575) -> ("亚硝酸盐跨度核查索引起始时间"=w576:string)
            }
            frame "硫化物" {
              n221 = Unbundle By Name(w578) -> ("硫化物跨度核查索引起始时间"=w577:string)
            }
            frame "ORP" {
              n222 = Unbundle By Name(w580) -> ("ORP跨度核查索引起始时间"=w579:string)
            }
            frame "", Default {
              n223 = global read "全局 时间2.vi" "跨度核查索引起始时间"() -> (w581:string)
            }
          }
        }
      }
      n224 = Get Date/Time In Seconds() -> (seconds since 1Jan1904=w428:timestamp)
      n225 = global read "断电保存全局.vi" "数据组合发送"() -> (w432:bool)
      n226 = Subtract(x=w428, y=w429) -> (x-y=w427:timestamp)
      n227 = Seconds To Date/Time(time stamp (now)=w427) -> (date time rec=w434:T7)  [unwired: 1 in]
      n228 = case shown="真" w432 {
        tunnel: w434 -> [w463 w468]
        tunnel: [w463 w467] -> w433
        tunnel: w420 -> [_ w465]
        frame False {
        }
        frame True {
          n229 = Equal?(x=w465, y="水样测试") -> (x = y?=w464:bool)
          n230 = case shown="真" w464 {
            tunnel: w468 -> [w469 w472]
            tunnel: [w469 w470] -> w467
            frame False {
            }
            frame True {
              # "水样测试延时2小时"
              n231 = Unbundle By Name(w472) -> ("时"=w474:i32)
              n232 = Subtract(x=w474, y=2) -> (x-y=w471:i32)
              n233 = Bundle By Name(cluster=w472, "时"=w471) -> (w470:T7)
            }
          }
        }
      }
      n234 = Date/Time To Seconds(2:w433) -> (0:w438:timestamp)  [unwired: 1 in]
      n235 = Format Date/Time String(time format string (%c)="%Y/%m/%d %H:%M:%S" ("时间格式字符串(%c)"), seconds (now)=w438) -> (date/time string=w436:string)  [unwired: 1 in]
      n236 = case shown="\"空白测试\", \"跨度核查\"" w420 {
        tunnel: [string[] ["时间", "测量模式", "数据类型", "检测值", "单位", "数据标识", "因子编码", "标样参考值"] ("columns") string[] ["时间", "测量模式", "数据类型", "检测值", "单位", "数据标识", "因子编码", "标样参考值", "跨度值"] ("columns")] -> w430
        frame "假", Default {
        }
        frame "空白测试", "跨度核查" {
        }
      }
      n237 = Format Into String(format string="#%s#" ("初始字符串"), w439) -> (resulting string=w444:string)  [unwired: 2 in, 1 out]
      n238 = Format Into String(format string="#%s#" ("初始字符串"), w436) -> (resulting string=w441:string)  [unwired: 2 in, 1 out]
      n239 = Concatenate Strings(w435, w444, "and 时间 < " ("字符串"), w441, " order by 时间 asc" ("字符串")) -> (w423:string)
      n240 = call "SQL查询.vi"("condition"=w423, "columns"=w430, "table输入"=w425, "database"=w424) -> ("error out"=w426:errorcluster, "data"=w422:string[][])  [unwired: 5 in, 1 out]
      n241 = case shown="错误" w426 {
        selector: w426 -> [w445 _]
        tunnel: w420 -> [_ w453]
        tunnel: w425 -> [_ w452]
        tunnel: w424 -> [_ w451]
        tunnel: w423 -> [_ w450]
        tunnel: w422 -> [w446 w448]
        tunnel: [w446 w449] -> w421
        tunnel: [w445 w447] -> w419
        frame No Error {
        }
        frame Error {
          # "兼容旧数据库没有跨度值版本"
          n242 = case shown="\"假\", 默认" w453 {
            tunnel: w452 -> [_ w459]
            tunnel: w451 -> [_ w458]
            tunnel: w450 -> [_ w457]
            tunnel: [w454 w456] -> w449
            tunnel: w448 -> [w454 _]
            tunnel: [_ w455] -> w447
            frame "假", Default {
            }
            frame "空白测试", "跨度核查" {
              n243 = call "SQL查询.vi"("condition"=w457, "columns"=string[] ["时间", "测量模式", "数据类型", "检测值", "单位", "数据标识", "因子编码", "标样参考值"], "table输入"=w459, "database"=w458) -> ("error out"=w455:errorcluster, "data"=w456:string[][])  [unwired: 5 in, 1 out]
            }
          }
        }
      }
      n244 = case shown="默认" w425 {
        tunnel: w425 -> [_ w584]
        tunnel: w423 -> [_ w583]
        tunnel: w421 -> [_ w582]
        frame Default {
        }
        frame "CODCr", "总氮", "总磷" {
          n245 = global write "全局 实时数据参数.vi" "data"(w582) -> ()
          n246 = global write "全局 实时数据参数.vi" "参数"(w584) -> ()
          n247 = global write "全局 实时数据参数.vi" "连接的字符串"(w583) -> ()
        }
      }
    }
    frame "加标回收" {
      w595 = "加标回收率" ("字符串")
      # "上传加标回收数据"
      n248 = global read "全局 数据发送重叠.vi" "掉线指示灯"() -> (w596:bool)
      n249 = case shown="假" w596 {
        tunnel: [w612 w626] -> w597
        frame False {
          n250 = global read "全局 时间2.vi" "加标回收索引"() -> (w618:T8)
          n251 = Unbundle By Name(w618) -> ("氨氮加标回收索引起始时间"=w617:string, "总磷加标回收索引起始时间"=w616:string, "总氮加标回收索引起始时间"=w615:string, "CODMn加标回收索引起始时间"=w614:string, "CODCr加标回收索引起始时间"=w613:string)
          n252 = local read "查询元素输入"() -> (w619:string)
          n253 = case shown="\"\", 默认" w619 {
            tunnel: [w620 w621 w622 w623 w624 w625] -> w612
            tunnel: w617 -> [_ _ w622 _ _ _]
            tunnel: w616 -> [_ _ _ w623 _ _]
            tunnel: w615 -> [_ _ _ _ w624 _]
            tunnel: w614 -> [w620 _ _ _ _ _]
            tunnel: w613 -> [_ w621 _ _ _ _]
            frame "CODMn加标回收率" {
            }
            frame "CODCr加标回收率" {
            }
            frame "氨氮加标回收率" {
            }
            frame "总磷加标回收率" {
            }
            frame "总氮加标回收率" {
            }
            frame "", Default {
              n254 = global read "全局 时间2.vi" "加标回收索引起始时间"() -> (w625:string)
            }
          }
        }
        frame True {
          n255 = global read "全局 数据发送重叠.vi" "TCP掉线时间节点"() -> (w626:string)
        }
      }
      n256 = global read "断电保存全局.vi" "数据发送延时时间/s"() -> (w587:i32)
      n257 = Get Date/Time In Seconds() -> (seconds since 1Jan1904=w586:timestamp)
      n258 = Subtract(x=w586, y=w587) -> (x-y=w585:timestamp)
      n259 = Seconds To Date/Time(time stamp (now)=w585) -> (date time rec=w592:T7)  [unwired: 1 in]
      n260 = Date/Time To Seconds(2:w592) -> (0:w594:timestamp)  [unwired: 1 in]
      n261 = Format Date/Time String(time format string (%c)="%Y/%m/%d %H:%M:%S" ("时间格式字符串(%c)"), seconds (now)=w594) -> (date/time string=w591:string)  [unwired: 1 in]
      n262 = Format Into String(format string="#%s#" ("初始字符串"), w597) -> (resulting string=w611:string)  [unwired: 2 in, 1 out]
      n263 = Format Into String(format string="#%s#" ("初始字符串"), w591) -> (resulting string=w607:string)  [unwired: 2 in, 1 out]
      n264 = Concatenate Strings("where 参数 ='" ("condition"), w590, "' and 时间 > ", w611, "and 时间 < " ("字符串"), w607, " order by 时间 asc" ("字符串")) -> (w599:string)
      n265 = call "SQL查询.vi"("condition"=w599, "columns"=string[] ["时间", "参数", "加标前水样测试时间", "加标前水样浓度值", "加标后水样浓度值", "加标母液浓度值", "加标体积", "加标水杯定容体积", "加标回收率"], "table输入"=w595, "database"="database1.mdb") -> ("error out"=w601:errorcluster, "data"=w598:string[][])  [unwired: 5 in, 1 out]
      n266 = case shown="\"CODCr\", \"总氮\", \"总磷\"" w595 {
        tunnel: w595 -> [_ w629]
        tunnel: w599 -> [_ w628]
        tunnel: w598 -> [_ w627]
        frame Default {
        }
        frame "CODCr", "总氮", "总磷" {
          n267 = global write "全局 实时数据参数.vi" "data"(w627) -> ()
          n268 = global write "全局 实时数据参数.vi" "参数"(w629) -> ()
          n269 = global write "全局 实时数据参数.vi" "连接的字符串"(w628) -> ()
        }
      }
      n270 = case shown="假" FALSE {
        tunnel: [w631 w634] -> w603
        tunnel: w598 -> [w631 w633]
        tunnel: w601 -> [w630 w632]
        tunnel: [w630 w632] -> w600
        frame False {
        }
        frame True {
          # "数字字符串精度转换保留"
          n271 = Index Array(array=w633, index (col)=3 ("禁用的索引 (列)")) -> (element=w640:string[])  [unwired: 1 in]
          n272 = for {
            tunnel: w640 -> [w643] mode=indexing
            tunnel: [w642] -> w636 mode=indexing
            n273 = Fract/Exp String To Number(string=w643) -> (number=w644:dbl)  [unwired: 3 in, 1 out]
            n274 = Number To Fractional String(number=w644, precision (6)=i16 2 ("精度(6)")) -> (F-format string=w642:string)  [unwired: 2 in]
          }
          n275 = Delete From Array(array=w633, length=1 ("长度"), index (col)=3 ("禁用的索引 (列)")) -> (array with subset deleted=w637:string[][])  [unwired: 1 in, 1 out]
          n276 = Insert Into Array(array=w637, index (col)=3 ("禁用的索引 (列)"), new element=w636) -> (w634:string[][])  [unwired: 1 in]
        }
      }
    }
    frame "平行样测试" {
      w656 = "平行样测试" ("字符串")
      # "上传本地时间点的实时数据"
      # "上传平行样数据"
      n277 = global read "全局 数据发送重叠.vi" "掉线指示灯"() -> (w657:bool)
      n278 = case shown="假" w657 {
        tunnel: [w680 w687] -> w658
        frame False {
          n279 = global read "全局 时间2.vi" "平行样索引"() -> (w678:T9)
          n280 = Unbundle By Name(w678) -> ("氨氮平行样索引起始时间"=w677:string, "总磷平行样索引起始时间"=w676:string, "总氮平行样索引起始时间"=w675:string, "CODMn平行样索引起始时间"=w674:string, "CODCr平行样索引起始时间"=w673:string)
          n281 = local read "查询元素输入"() -> (w679:string)
          n282 = case shown="\"CODCr\"" w679 {
            tunnel: [w681 w682 w683 w684 w685 w686] -> w680
            tunnel: w677 -> [_ _ w683 _ _ _]
            tunnel: w676 -> [_ _ _ w684 _ _]
            tunnel: w675 -> [_ _ _ _ w685 _]
            tunnel: w674 -> [w681 _ _ _ _ _]
            tunnel: w673 -> [_ w682 _ _ _ _]
            frame "CODMn" {
            }
            frame "CODCr" {
            }
            frame "氨氮" {
            }
            frame "总磷" {
            }
            frame "总氮" {
            }
            frame "", Default {
              n283 = global read "全局 时间2.vi" "平行样索引起始时间"() -> (w686:string)
            }
          }
        }
        frame True {
          n284 = global read "全局 数据发送重叠.vi" "TCP掉线时间节点"() -> (w687:string)
        }
      }
      n285 = global read "断电保存全局.vi" "数据发送延时时间/s"() -> (w648:i32)
      n286 = Get Date/Time In Seconds() -> (seconds since 1Jan1904=w647:timestamp)
      n287 = Subtract(x=w647, y=w648) -> (x-y=w646:timestamp)
      n288 = Seconds To Date/Time(time stamp (now)=w646) -> (date time rec=w653:T7)  [unwired: 1 in]
      n289 = Date/Time To Seconds(2:w653) -> (0:w655:timestamp)  [unwired: 1 in]
      n290 = Format Date/Time String(time format string (%c)="%Y/%m/%d %H:%M:%S" ("时间格式字符串(%c)"), seconds (now)=w655) -> (date/time string=w652:string)  [unwired: 1 in]
      n291 = Format Into String(format string="#%s#" ("初始字符串"), w658) -> (resulting string=w672:string)  [unwired: 2 in, 1 out]
      n292 = Format Into String(format string="#%s#" ("初始字符串"), w652) -> (resulting string=w668:string)  [unwired: 2 in, 1 out]
      n293 = Concatenate Strings("where 参数 ='" ("condition"), w651, "' and 时间 > ", w672, "and 时间 < " ("字符串"), w668, " order by 时间 asc" ("字符串")) -> (w660:string)
      n294 = call "SQL查询.vi"("condition"=w660, "columns"=string[] ["时间", "参数", "第一次水样浓度值", "第二次水样测试时间", "第二次水样浓度值"], "table输入"=w656, "database"="database1.mdb") -> ("error out"=w662:errorcluster, "data"=w659:string[][])  [unwired: 5 in, 1 out]
      n295 = case shown="默认" w656 {
        tunnel: w656 -> [_ w690]
        tunnel: w660 -> [_ w689]
        tunnel: w659 -> [_ w688]
        frame Default {
        }
        frame "CODCr", "总氮", "总磷" {
          n296 = global write "全局 实时数据参数.vi" "data"(w688) -> ()
          n297 = global write "全局 实时数据参数.vi" "参数"(w690) -> ()
          n298 = global write "全局 实时数据参数.vi" "连接的字符串"(w689) -> ()
        }
      }
      n299 = case shown="假" FALSE {
        tunnel: [w692 w695] -> w664
        tunnel: w659 -> [w692 w694]
        tunnel: w662 -> [w691 w693]
        tunnel: [w691 w693] -> w661
        frame False {
        }
        frame True {
          # "数字字符串精度转换保留"
          n300 = Index Array(array=w694, index (col)=3 ("禁用的索引 (列)")) -> (element=w701:string[])  [unwired: 1 in]
          n301 = for {
            tunnel: w701 -> [w704] mode=indexing
            tunnel: [w703] -> w697 mode=indexing
            n302 = Fract/Exp String To Number(string=w704) -> (number=w705:dbl)  [unwired: 3 in, 1 out]
            n303 = Number To Fractional String(number=w705, precision (6)=i16 2 ("精度(6)")) -> (F-format string=w703:string)  [unwired: 2 in]
          }
          n304 = Delete From Array(array=w694, length=1 ("长度"), index (col)=3 ("禁用的索引 (列)")) -> (array with subset deleted=w698:string[][])  [unwired: 1 in, 1 out]
          n305 = Insert Into Array(array=w698, index (col)=3 ("禁用的索引 (列)"), new element=w697) -> (w695:string[][])  [unwired: 1 in]
        }
      }
    }
    frame "集成干预测试" {
      # "上传本地时间点的实时数据"
      # "上传集成干预数据"
      n306 = global read "断电保存全局.vi" "应用环境"() -> (w711:enum16{"STD", "GB212"})
      n307 = case shown="\"GB212\"" w711 {
        tunnel: w710 -> [w733 w741]
        tunnel: ["集成干预测试" ("字符串") w741] -> w709
        tunnel: [string[] ["时间", "参数", "集成干预测试浓度值", "集成干预前测试时间", "集成干预前测试浓度值"] ("columns") string[] ["时间", "测量模式", "数据类型", "检测值", "单位", "数据标识", "因子编码", "标样参考值"] ("columns")] -> w708
        tunnel: [w734 w740] -> w707
        frame "STD", Default {
          n308 = Concatenate Strings("where 参数 ='" ("condition"), w733) -> (w734:string)
        }
        frame "GB212" {
          n309 = Concatenate Strings("where 测量模式 ='" ("condition"), "集成干预测试" ("字符串")) -> (w740:string)
        }
      }
      n310 = global read "全局 数据发送重叠.vi" "掉线指示灯"() -> (w720:bool)
      n311 = case shown="假" w720 {
        tunnel: [w742 w776] -> w721
        frame False {
          n312 = local read "查询元素输入"() -> (w743:string)
          n313 = global read "全局 时间2.vi" "集成干预索引"() -> (w744:T10)
          n314 = case shown="\"CODMn\"" w743 {
            tunnel: [w745 w747 w749 w751 w753 w755 w757 w759 w761 w763 w765 w767 w769 w771 w773 w775] -> w742
            tunnel: w744 -> [w746 w748 w750 w752 w754 w756 w758 w760 w762 w764 w766 w768 w770 w772 w774 _]
            frame "CODMn" {
              n315 = Unbundle By Name(w746) -> ("CODMn集成干预索引起始时间"=w745:string)
            }
            frame "CODCr" {
              n316 = Unbundle By Name(w748) -> ("CODCr集成干预索引起始时间"=w747:string)
            }
            frame "氨氮" {
              n317 = Unbundle By Name(w750) -> ("氨氮集成干预索引起始时间"=w749:string)
            }
            frame "总磷" {
              n318 = Unbundle By Name(w752) -> ("总磷集成干预索引起始时间"=w751:string)
            }
            frame "总氮" {
              n319 = Unbundle By Name(w754) -> ("总氮集成干预索引起始时间"=w753:string)
            }
            frame "DO" {
              n320 = Unbundle By Name(w756) -> ("DO集成干预索引起始时间"=w755:string)
            }
            frame "PH" {
              n321 = Unbundle By Name(w758) -> ("PH集成干预索引起始时间"=w757:string)
            }
            frame "比电导率" {
              n322 = Unbundle By Name(w760) -> ("比电导率集成干预索引起始时间"=w759:string)
            }
            frame "水温" {
              n323 = Unbundle By Name(w762) -> ("水温集成干预索引起始时间"=w761:string)
            }
            frame "浊度" {
              n324 = Unbundle By Name(w764) -> ("浊度集成干预索引起始时间"=w763:string)
            }
            frame "叶绿素a" {
              n325 = Unbundle By Name(w766) -> ("叶绿素a集成干预索引起始时间"=w765:string)
            }
            frame "藻密度" {
              n326 = Unbundle By Name(w768) -> ("藻密度集成干预索引起始时间"=w767:string)
            }
            frame "亚硝酸盐" {
              n327 = Unbundle By Name(w770) -> ("亚硝酸盐集成干预索引起始时间"=w769:string)
            }
            frame "硫化物" {
              n328 = Unbundle By Name(w772) -> ("硫化物集成干预索引起始时间"=w771:string)
            }
            frame "ORP" {
              n329 = Unbundle By Name(w774) -> ("ORP集成干预索引起始时间"=w773:string)
            }
            frame "", Default {
              n330 = global read "全局 时间2.vi" "平行样索引起始时间"() -> (w775:string)
            }
          }
        }
        frame True {
          n331 = global read "全局 数据发送重叠.vi" "TCP掉线时间节点"() -> (w776:string)
        }
      }
      n332 = global read "断电保存全局.vi" "数据发送延时时间/s"() -> (w714:i32)
      n333 = Get Date/Time In Seconds() -> (seconds since 1Jan1904=w713:timestamp)
      n334 = Subtract(x=w713, y=w714) -> (x-y=w712:timestamp)
      n335 = Seconds To Date/Time(time stamp (now)=w712) -> (date time rec=w717:T7)  [unwired: 1 in]
      n336 = Date/Time To Seconds(2:w717) -> (0:w719:timestamp)  [unwired: 1 in]
      n337 = Format Date/Time String(time format string (%c)="%Y/%m/%d %H:%M:%S" ("时间格式字符串(%c)"), seconds (now)=w719) -> (date/time string=w716:string)  [unwired: 1 in]
      n338 = Format Into String(format string="#%s#" ("初始字符串"), w721) -> (resulting string=w731:string)  [unwired: 2 in, 1 out]
      n339 = Format Into String(format string="#%s#" ("初始字符串"), w716) -> (resulting string=w727:string)  [unwired: 2 in, 1 out]
      n340 = Concatenate Strings(w707, "' and 时间 > ", w731, "and 时间 < " ("字符串"), w727, " order by 时间 asc" ("字符串")) -> (w723:string)
      n341 = call "SQL查询.vi"("condition"=w723, "columns"=w708, "table输入"=w709, "database"="database1.mdb") -> ("error out"=w724:errorcluster, "data"=w722:string[][])  [unwired: 5 in, 1 out]
      n342 = case shown="\"CODCr\", \"总氮\", \"总磷\"" w709 {
        tunnel: w709 -> [_ w779]
        tunnel: w723 -> [_ w778]
        tunnel: w722 -> [_ w777]
        frame Default {
        }
        frame "CODCr", "总氮", "总磷" {
          n343 = global write "全局 实时数据参数.vi" "data"(w777) -> ()
          n344 = global write "全局 实时数据参数.vi" "参数"(w779) -> ()
          n345 = global write "全局 实时数据参数.vi" "连接的字符串"(w778) -> ()
        }
      }
    }
    frame "提取加标回收" {
      w783 = "加标回收率" ("字符串")
      # "上传本地时间点的实时数据"
      n346 = global read "全局 数据发送重叠.vi" "掉线指示灯"() -> (w784:bool)
      n347 = case shown="假" w784 {
        tunnel: [w800 w801] -> w785
        frame False {
          n348 = global read "起始时间.vi" "起始时间"() -> (w800:string)
        }
        frame True {
          n349 = global read "全局 数据发送重叠.vi" "TCP掉线时间节点"() -> (w801:string)
        }
      }
      n350 = global read "起始时间.vi" "结束时间"() -> (w782:string)
      n351 = Format Into String(format string="#%s#" ("初始字符串"), w785) -> (resulting string=w799:string)  [unwired: 2 in, 1 out]
      n352 = Format Into String(format string="#%s#" ("初始字符串"), w782) -> (resulting string=w795:string)  [unwired: 2 in, 1 out]
      n353 = Concatenate Strings("where 参数 ='" ("condition"), w781, "' and 时间 between ", w799, "and" ("字符串"), w795) -> (w787:string)
      n354 = call "SQL查询.vi"("condition"=w787, "columns"=string[] ["时间", "参数", "加标前水样测试时间", "加标前水样浓度值", "加标后水样浓度值", "加标母液浓度值", "加标体积", "加标水杯定容体积", "加标回收率"], "table输入"=w783, "database"="database1.mdb") -> ("error out"=w789:errorcluster, "data"=w786:string[][])  [unwired: 5 in, 1 out]
      n355 = case shown="\"CODCr\", \"总氮\", \"总磷\"" w783 {
        tunnel: w783 -> [_ w804]
        tunnel: w787 -> [_ w803]
        tunnel: w786 -> [_ w802]
        frame Default {
        }
        frame "CODCr", "总氮", "总磷" {
          n356 = global write "全局 实时数据参数.vi" "data"(w802) -> ()
          n357 = global write "全局 实时数据参数.vi" "参数"(w804) -> ()
          n358 = global write "全局 实时数据参数.vi" "连接的字符串"(w803) -> ()
        }
      }
      n359 = case shown="假" FALSE {
        tunnel: [w806 w809] -> w791
        tunnel: w786 -> [w806 w808]
        tunnel: w789 -> [w805 w807]
        tunnel: [w805 w807] -> w788
        frame False {
        }
        frame True {
          # "数字字符串精度转换保留"
          n360 = Index Array(array=w808, index (col)=3 ("禁用的索引 (列)")) -> (element=w815:string[])  [unwired: 1 in]
          n361 = for {
            tunnel: w815 -> [w818] mode=indexing
            tunnel: [w817] -> w811 mode=indexing
            n362 = Fract/Exp String To Number(string=w818) -> (number=w819:dbl)  [unwired: 3 in, 1 out]
            n363 = Number To Fractional String(number=w819, precision (6)=i16 2 ("精度(6)")) -> (F-format string=w817:string)  [unwired: 2 in]
          }
          n364 = Delete From Array(array=w808, length=1 ("长度"), index (col)=3 ("禁用的索引 (列)")) -> (array with subset deleted=w812:string[][])  [unwired: 1 in, 1 out]
          n365 = Insert Into Array(array=w812, index (col)=3 ("禁用的索引 (列)"), new element=w811) -> (w809:string[][])  [unwired: 1 in]
        }
      }
    }
    frame "提取平行样" {
      w824 = "平行样测试" ("字符串")
      # "上传本地时间点的实时数据"
      n366 = global read "全局 数据发送重叠.vi" "掉线指示灯"() -> (w825:bool)
      n367 = case shown="假" w825 {
        tunnel: [w841 w842] -> w826
        frame False {
          n368 = global read "起始时间.vi" "起始时间"() -> (w841:string)
        }
        frame True {
          n369 = global read "全局 数据发送重叠.vi" "TCP掉线时间节点"() -> (w842:string)
        }
      }
      n370 = global read "起始时间.vi" "结束时间"() -> (w823:string)
      n371 = Format Into String(format string="#%s#" ("初始字符串"), w826) -> (resulting string=w840:string)  [unwired: 2 in, 1 out]
      n372 = Format Into String(format string="#%s#" ("初始字符串"), w823) -> (resulting string=w836:string)  [unwired: 2 in, 1 out]
      n373 = Concatenate Strings("where 参数 ='" ("condition"), w822, "' and 时间 between ", w840, "and" ("字符串"), w836) -> (w828:string)
      n374 = call "SQL查询.vi"("condition"=w828, "columns"=string[] ["时间", "参数", "第一次水样浓度值", "第二次水样测试时间", "第二次水样浓度值"], "table输入"=w824, "database"="database1.mdb") -> ("error out"=w830:errorcluster, "data"=w827:string[][])  [unwired: 5 in, 1 out]
      n375 = case shown="\"CODCr\", \"总氮\", \"总磷\"" w824 {
        tunnel: w824 -> [_ w845]
        tunnel: w828 -> [_ w844]
        tunnel: w827 -> [_ w843]
        frame Default {
        }
        frame "CODCr", "总氮", "总磷" {
          n376 = global write "全局 实时数据参数.vi" "data"(w843) -> ()
          n377 = global write "全局 实时数据参数.vi" "参数"(w845) -> ()
          n378 = global write "全局 实时数据参数.vi" "连接的字符串"(w844) -> ()
        }
      }
      n379 = case shown="假" FALSE {
        tunnel: [w847 w850] -> w832
        tunnel: w827 -> [w847 w849]
        tunnel: w830 -> [w846 w848]
        tunnel: [w846 w848] -> w829
        frame False {
        }
        frame True {
          # "数字字符串精度转换保留"
          n380 = Index Array(array=w849, index (col)=3 ("禁用的索引 (列)")) -> (element=w856:string[])  [unwired: 1 in]
          n381 = for {
            tunnel: w856 -> [w859] mode=indexing
            tunnel: [w858] -> w852 mode=indexing
            n382 = Fract/Exp String To Number(string=w859) -> (number=w860:dbl)  [unwired: 3 in, 1 out]
            n383 = Number To Fractional String(number=w860, precision (6)=i16 2 ("精度(6)")) -> (F-format string=w858:string)  [unwired: 2 in]
          }
          n384 = Delete From Array(array=w849, length=1 ("长度"), index (col)=3 ("禁用的索引 (列)")) -> (array with subset deleted=w853:string[][])  [unwired: 1 in, 1 out]
          n385 = Insert Into Array(array=w853, index (col)=3 ("禁用的索引 (列)"), new element=w852) -> (w850:string[][])  [unwired: 1 in]
        }
      }
    }
    frame "提取集成干预" {
      # "上传本地时间点的实时数据"
      n386 = global read "断电保存全局.vi" "应用环境"() -> (w866:enum16{"STD", "GB212"})
      n387 = case shown="\"GB212\"" w866 {
        tunnel: w862 -> [w884 w892]
        tunnel: ["集成干预测试" ("字符串") w892] -> w864
        tunnel: [string[] ["时间", "参数", "集成干预测试浓度值", "集成干预前测试时间", "集成干预前测试浓度值"] ("columns") string[] ["时间", "测量模式", "数据类型", "检测值", "单位", "数据标识", "因子编码", "标样参考值"] ("columns")] -> w865
        tunnel: [w885 w891] -> w863
        frame "STD", Default {
          n388 = Concatenate Strings("where 参数 ='" ("condition"), w884) -> (w885:string)
        }
        frame "GB212" {
          n389 = Concatenate Strings("where 测量模式 ='" ("condition"), "集成干预测试" ("字符串")) -> (w891:string)
        }
      }
      n390 = global read "全局 数据发送重叠.vi" "掉线指示灯"() -> (w868:bool)
      n391 = case shown="假" w868 {
        tunnel: [w893 w894] -> w869
        frame False {
          n392 = global read "起始时间.vi" "起始时间"() -> (w893:string)
        }
        frame True {
          n393 = global read "全局 数据发送重叠.vi" "TCP掉线时间节点"() -> (w894:string)
        }
      }
      n394 = global read "起始时间.vi" "结束时间"() -> (w867:string)
      n395 = Format Into String(format string="#%s#" ("初始字符串"), w869) -> (resulting string=w882:string)  [unwired: 2 in, 1 out]
      n396 = Format Into String(format string="#%s#" ("初始字符串"), w867) -> (resulting string=w878:string)  [unwired: 2 in, 1 out]
      n397 = Concatenate Strings(w863, "' and 时间 between ", w882, "and" ("字符串"), w878) -> (w871:string)
      n398 = call "SQL查询.vi"("condition"=w871, "columns"=w865, "table输入"=w864, "database"="database1.mdb") -> ("error out"=w873:errorcluster, "data"=w870:string[][])  [unwired: 5 in, 1 out]
      n399 = case shown="\"CODCr\", \"总氮\", \"总磷\"" w864 {
        tunnel: w864 -> [_ w897]
        tunnel: w871 -> [_ w896]
        tunnel: w870 -> [_ w895]
        frame Default {
        }
        frame "CODCr", "总氮", "总磷" {
          n400 = global write "全局 实时数据参数.vi" "data"(w895) -> ()
          n401 = global write "全局 实时数据参数.vi" "参数"(w897) -> ()
          n402 = global write "全局 实时数据参数.vi" "连接的字符串"(w896) -> ()
        }
      }
      n403 = case shown="假" FALSE {
        tunnel: [w899 w902] -> w875
        tunnel: w870 -> [w899 w901]
        tunnel: w873 -> [w898 w900]
        tunnel: [w898 w900] -> w872
        frame False {
        }
        frame True {
          # "数字字符串精度转换保留"
          n404 = Index Array(array=w901, index (col)=3 ("禁用的索引 (列)")) -> (element=w908:string[])  [unwired: 1 in]
          n405 = for {
            tunnel: w908 -> [w911] mode=indexing
            tunnel: [w910] -> w904 mode=indexing
            n406 = Fract/Exp String To Number(string=w911) -> (number=w912:dbl)  [unwired: 3 in, 1 out]
            n407 = Number To Fractional String(number=w912, precision (6)=i16 2 ("精度(6)")) -> (F-format string=w910:string)  [unwired: 2 in]
          }
          n408 = Delete From Array(array=w901, length=1 ("长度"), index (col)=3 ("禁用的索引 (列)")) -> (array with subset deleted=w905:string[][])  [unwired: 1 in, 1 out]
          n409 = Insert Into Array(array=w905, index (col)=3 ("禁用的索引 (列)"), new element=w904) -> (w902:string[][])  [unwired: 1 in]
        }
      }
    }
    frame "提取实时数据" {
      # "上传给定时间段之间的实时数据"
      n410 = global read "起始时间.vi" "起始时间"() -> (w925:string)
      n411 = global read "起始时间.vi" "结束时间"() -> (w924:string)
      n412 = global read "全局 实时数据参数.vi" "实时数据参数"() -> (w914:string)
      n413 = Format Into String(format string="#%s#" ("初始字符串"), w925) -> (resulting string=w932:string)  [unwired: 2 in, 1 out]
      n414 = Format Into String(format string="#%s#" ("初始字符串"), w924) -> (resulting string=w926:string)  [unwired: 2 in, 1 out]
      n415 = Concatenate Strings("where 测量模式 ='" ("condition"), w914, "' and 时间 between ", w932, "and" ("字符串"), w926) -> (w930:string)
      n416 = call "SQL查询.vi"("condition"=w930, "columns"=string[] ["时间", "测量模式", "数据类型", "检测值", "单位", "数据标识", "因子编码", "标样参考值"], "table输入"=w916, "database"="database1.mdb") -> ("error out"=w921:errorcluster, "data"=w923:string[][])  [unwired: 5 in, 1 out]
      n417 = case shown="假" FALSE {
        tunnel: w923 -> [w934 w942]
        tunnel: [w934 w936] -> w922
        tunnel: w921 -> [w933 w935]
        tunnel: [w933 w935] -> w920
        frame False {
        }
        frame True {
          # "数字字符串精度转换保留"
          n418 = Index Array(array=w942, index (col)=3 ("禁用的索引 (列)")) -> (element=w943:string[])  [unwired: 1 in]
          n419 = for {
            tunnel: w943 -> [w946] mode=indexing
            tunnel: [w945] -> w938 mode=indexing
            n420 = Fract/Exp String To Number(string=w946) -> (number=w947:dbl)  [unwired: 3 in, 1 out]
            n421 = Number To Fractional String(number=w947, precision (6)=i16 2 ("精度(6)")) -> (F-format string=w945:string)  [unwired: 2 in]
          }
          n422 = Delete From Array(array=w942, length=1 ("长度"), index (col)=3 ("禁用的索引 (列)")) -> (array with subset deleted=w939:string[][])  [unwired: 1 in, 1 out]
          n423 = Insert Into Array(array=w939, index (col)=3 ("禁用的索引 (列)"), new element=w938) -> (w936:string[][])  [unwired: 1 in]
        }
      }
    }
  }
  "待发送数据" <- w4
  "columns输出" <- w1
  n424 = call <vilib>:"Clear Errors.vi"("error in (no error)"=w8) -> ("error out"=→"error out":errorcluster)  [unwired: 5 in, 1 out]
  n425 = Index Array(array=w4, index (row)=0 ("索引 (行)")) -> (element=→"待发送第一条数据":string[])  [unwired: 1 in]
